vi "Text control 2 v3.4.vi"() -> ()   [LabVIEW 2016]
panel:
  out "I vs Vd":cluster{"Y data in":dbl[], "X data in":dbl[]}[](graph)
  in  "Auto Reset":bool
  in  "Reset":bool
  out "Id min vs time":cluster{"Y data in":dbl[], "X data in":dbl[]}[](graph)
  in  "Time Offset":dbl caption="Set Start Time (s)"
  out "Total lines":i32
  out "Line running":i32
  in  "byte count":u32=64
  in  "Serial End Mode for Reads":u16(ring)=2 items=["None", "LastBit", "TermChar"]
  in  "Timeout (ms)":u32=10000
  in  "Enable Termination\nChar (T)":bool=TRUE
  in  "Termination char\n(0xA = '\\n' = LF)\n(0xD = '\\r' = CR)":u8=13 format="%.0x"
  in  "flow control":u16(ring) items=["None"=0, "XON/XOFF"=1, "RTS/CTS"=2, "DTR/DSR"=4]
  in  "stop bits":u16(ring)=10 items=["1.0"=10, "1.5"=15, "2.0"=20]
  in  "parity":u16(ring) items=["None", "Odd", "Even", "Mark", "Space"]
  in  "data bits":u16=8 min=5 max=8 step=1
  in  "VISA resource name":refnum<visa-resource-name>="COM6"
  in  "baud rate":u32=9600
  out "Serial port output":string
  out "error out":errorcluster
  in  "Units":u16(ring) items=["Seconds", "Minutes", "Hours"]
  out "Elapsed Time":dbl caption="Elapsed Time (s)"
  out "Id max vs time":cluster{"Y data in":dbl[], "X data in":dbl[]}[](graph)
  out "Ig":dbl format="%.2e"
  out "Id":dbl format="%.2e"
  out "Is":dbl format="%.2e"
  out "I vs Vg":cluster{"Y data in":dbl[], "X data in":dbl[]}[](graph)
  in  "Panel Controls 2":T1={"Emergency Stop"=refnum, "TransGraph Max"=1e-05, "Text/Graph (text=false)"=TRUE, "TransGraph Min"=1e-11} {"TransGraph Min" format="%.2e"; "TransGraph Max" format="%.2e"}
  out "Command running:":string="#output s 0 0 0 -0.008 0.008 0.002"
  in  "Standby":T2
  in  "Full Reset":bool
  in  "SMU4":cluster{"on/off":bool, "Voltage":dbl} {"Voltage" min=-100.0 max=100.0 format="%.2f"}
  in  "Source/Drain Range":u8(slide)=6 max=11 scale=0.0..11.0
  in  "Source/Drain\nRange mode":u16(ring) items=["Auto", "Limited", "Fixed"]
  in  "Gate Range":u8(slide)=6 max=11 scale=0.0..11.0
  in  "Gate Range\nmode":u16(ring) items=["Auto", "Limited", "Fixed"]
  in  "Gate":T3={"Gate Start"=0.0, "Gate Stop"=2.0, "Gate Step (linear only)"=1.0, "Gate Compliance"=0.0001, "Gate PComp"=0.0, "Range mode"=0, "Range"=6} {"Range" max=11 scale=0.0..11.0; "Range mode" items=["Auto", "Limited", "Fixed"]; "Gate PComp" format="%^.2e"; "Gate Compliance" format="%^.2e"; "Gate Step (linear only)" format="%^.4e"; "Gate Stop" format="%^.4e"; "Gate Start" format="%^.4e"}
  in  "Drain 2":T4={"Drain Start"=0.0, "Drain Stop"=2.0, "Drain Compliance"=0.0001, "Drain Step"=1.0, "Drain PComp"=0.0, "Range mode"=0, "Range"=6} {"Range" max=11 scale=0.0..11.0; "Range mode" items=["Auto", "Limited", "Fixed"]; "Drain PComp" format="%^.2e"; "Drain Step" format="%^.4e"; "Drain Compliance" format="%^.2e"; "Drain Stop" format="%^.4e"; "Drain Start" format="%^.4e"}
  in  "Timings 2":T5={"integration time"=0, "Short/Long integration time"=0.00064, "hold time (sec)"=0.0, "delay time (sec)"=0.0, "Step Time (0 disables)"=0.0, "sweep method"=0, "Pulse period"=0.005, "Base voltage"=0.0, "Pulse width"=0.0005} {"Pulse width" min=0.0005 max=0.1 step=0.0001 format="%.4f"; "Base voltage" format="%^.4e"; "Pulse period" min=0.005 max=1.0 step=0.0001 format="%.4f"; "sweep method" items=["Continuous", "Pulsed"]; "Step Time (0 disables)" format="%.2f"; "delay time (sec)" format="%.4f"; "hold time (sec)" format="%.4f"; "Short/Long integration time" format="%^.0e"; "integration time" scale=0.0..2.0}
  in  "Panel Controls":T6={"Emergency Stop"=refnum, "TransGraph Max"=1e-05, "Text/Graph (text=false)"=TRUE} {"TransGraph Max" format="%.2e"}
  in  "Interrupt run":bool
  in  "Drain: Compliance":dbl=0.001 format="%.8f"
  in  "Gate: Compliance":dbl=0.001 format="%.8f"
  out "Path":path=path "C:/users/rlp38/09Apr2009LTtesting/test2.txt"
  in  "hold time /s":dbl format="%.2f"
  in  "delay time /s":dbl format="%.2f"
  in  "integration time":u32(slide) max=2 step=1 scale=0.0..2.0
  in  "Integration time (short)":dbl=0.0019 min=8e-05 max=0.0019 step=8e-05 format="%^.0e"
  in  "Integration time (long)":dbl=0.32 min=0.04 max=2.0 step=0.02 format="%.2f"
  in  "Step delay /s":dbl format="%.2f"
  in  "Program":string="#pulsedstressV d 0.03 20 0 0.5 0.0827 5\n#\n#itime s\n#gaterangemode l\n#drainrangemode l\n#pulsed on 0.05 0 0.02\n#transfer d 1 -1 -0.1 -1 -1 0\n#wait-min 1\n#transfer d 1 -1 -0.1 -1 -1 0\n#output d 0 -1 -0.5 0 -1 -0.1\n#transfer d -10 40 1 5 40 35\n#transfer d -10 40 1 5 40 35\n#output d 0 40 20 0 40 1\n#\n#\n#sample 1 0.008 221 6 0.003\n#samplei 400e-6 200 6 0.002 0.1\n#vsu2pulse -10 4\n#\n#stressV 0.016 0.03 2e-4 0.1e-3 11\n#stressI 220e-7 0.08 15\n#transfer s -1 1 0.5 -0.005 0.005 0.005\n#output s 0 0 0 -0.008 0.008 0.002\n"
  # "Serial port settings"
  # "Time"
  # "1\n2\n3\n4\n5\n6\n7\n8\n9\n10\n11\n12\n13\n14\n15\n16\n17\n18\n19\n20\n21\n22\n23\n24\n25"
  # "100 samples is approx 13s with medium integration"
  # "Syntax:\nitime [s|m|l]\ngaterangemode [a|l|f]\ndrainrangemode [a|l|f]\npulsed [on|off] PulsePeriod(sec) PulseBaseVoltage PulseONWidth(sec)\nstandby [on l off]\nwait NumMilliseconds\nwait-min NumMinutes\n# texthere = comment\ntransfer [s|d] VgStart VgStop VgStep VdStart VdStop VdStep\noutput [s|d] VgStart VgStop VgStep VdStart VdStop VdStep\nsample Vg Vd NumSamples Time(s) SampleInterval(s)\nsamplei Idg NumSamples Time(s) SampleInterval(s) VDGcompliance\n# if in doubt use SampleInterval(s) = 0.004\nstressV VG VD IGcompliance IDcompliance Duration(sec)\nstressI IDG VDGcompliance Duration(sec)\nvsu2pulse Bias Duration(s)\npulsedstressV [s|d] VEstop VgON VgOFF Period(s) PulseONwidth(s) Vd\nsample-fpp Vg Vd NumSamples Time\nresample-fpp Vg Vd\ntransfer-fpp [s|d] VgStart VgStop VgStep VdStart VdStop VdStep\noutput-fpp [s|d] VgStart VgStop VgStep VdStart VdStop VdStep\nserial SerialPortCommand"
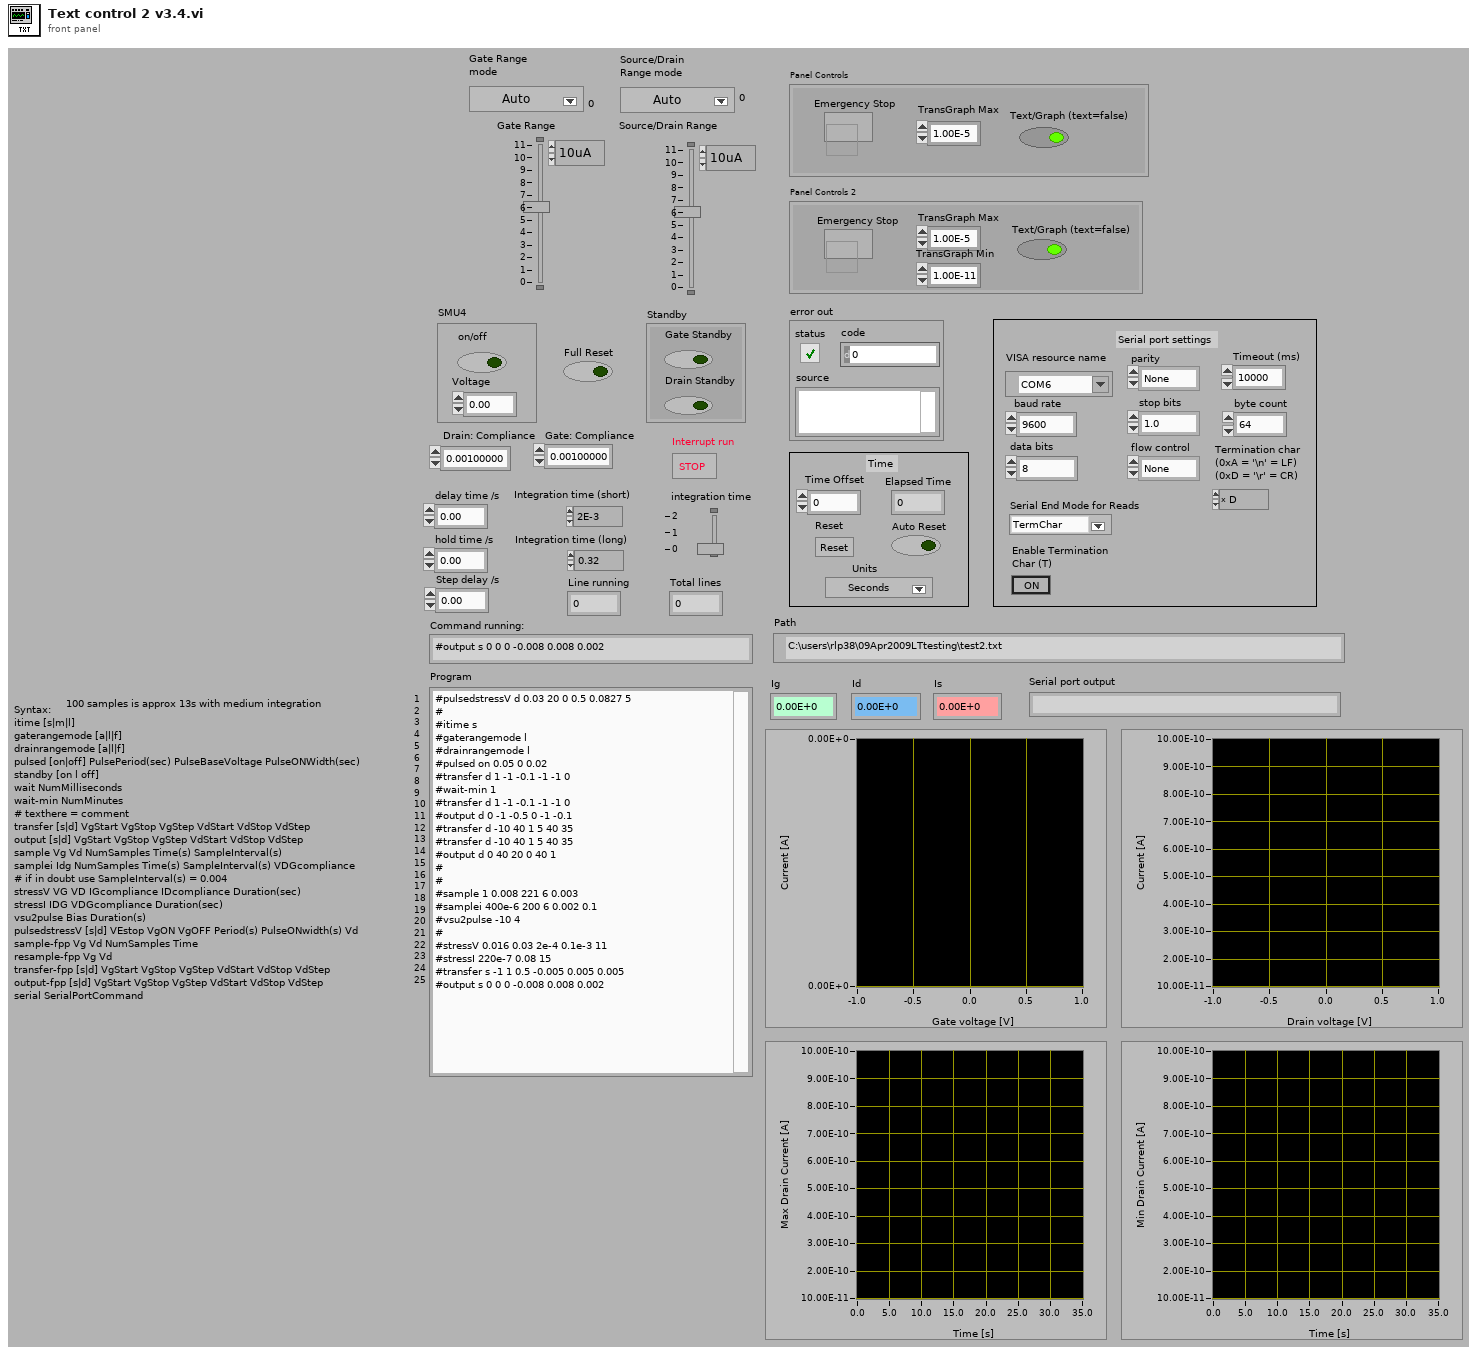
[diagram p1: front panel]
types:
  T1 = cluster{"Emergency Stop":refnum<vi>, "TransGraph Max":dbl, "Text/Graph (text=false)":bool, "TransGraph Min":dbl}
  T2 = cluster{"Gate Standby":bool, "Drain Standby":bool}
  T3 = cluster{"Gate Start":dbl, "Gate Stop":dbl, "Gate Step (linear only)":dbl, "Gate Compliance":dbl, "Gate PComp":dbl, "Range mode":u16, "Range":u8}
  T4 = cluster{"Drain Start":dbl, "Drain Stop":dbl, "Drain Compliance":dbl, "Drain Step":dbl, "Drain PComp":dbl, "Range mode":u16, "Range":u8}
  T5 = cluster{"integration time":u32, "Short/Long integration time":dbl, "hold time (sec)":dbl, "delay time (sec)":dbl, "Step Time (0 disables)":dbl, "sweep method":u16, "Pulse period":dbl, "Base voltage":dbl, "Pulse width":dbl}
  T6 = cluster{"Emergency Stop":refnum<vi>, "TransGraph Max":dbl, "Text/Graph (text=false)":bool}
  T7 = enum16{"open", "replace", "create", "open or create", "replace or create", "replace or create with confirmation"}
  T8 = cluster{"V2 Start":dbl, "V2 Step":dbl, "Number of points":i32}
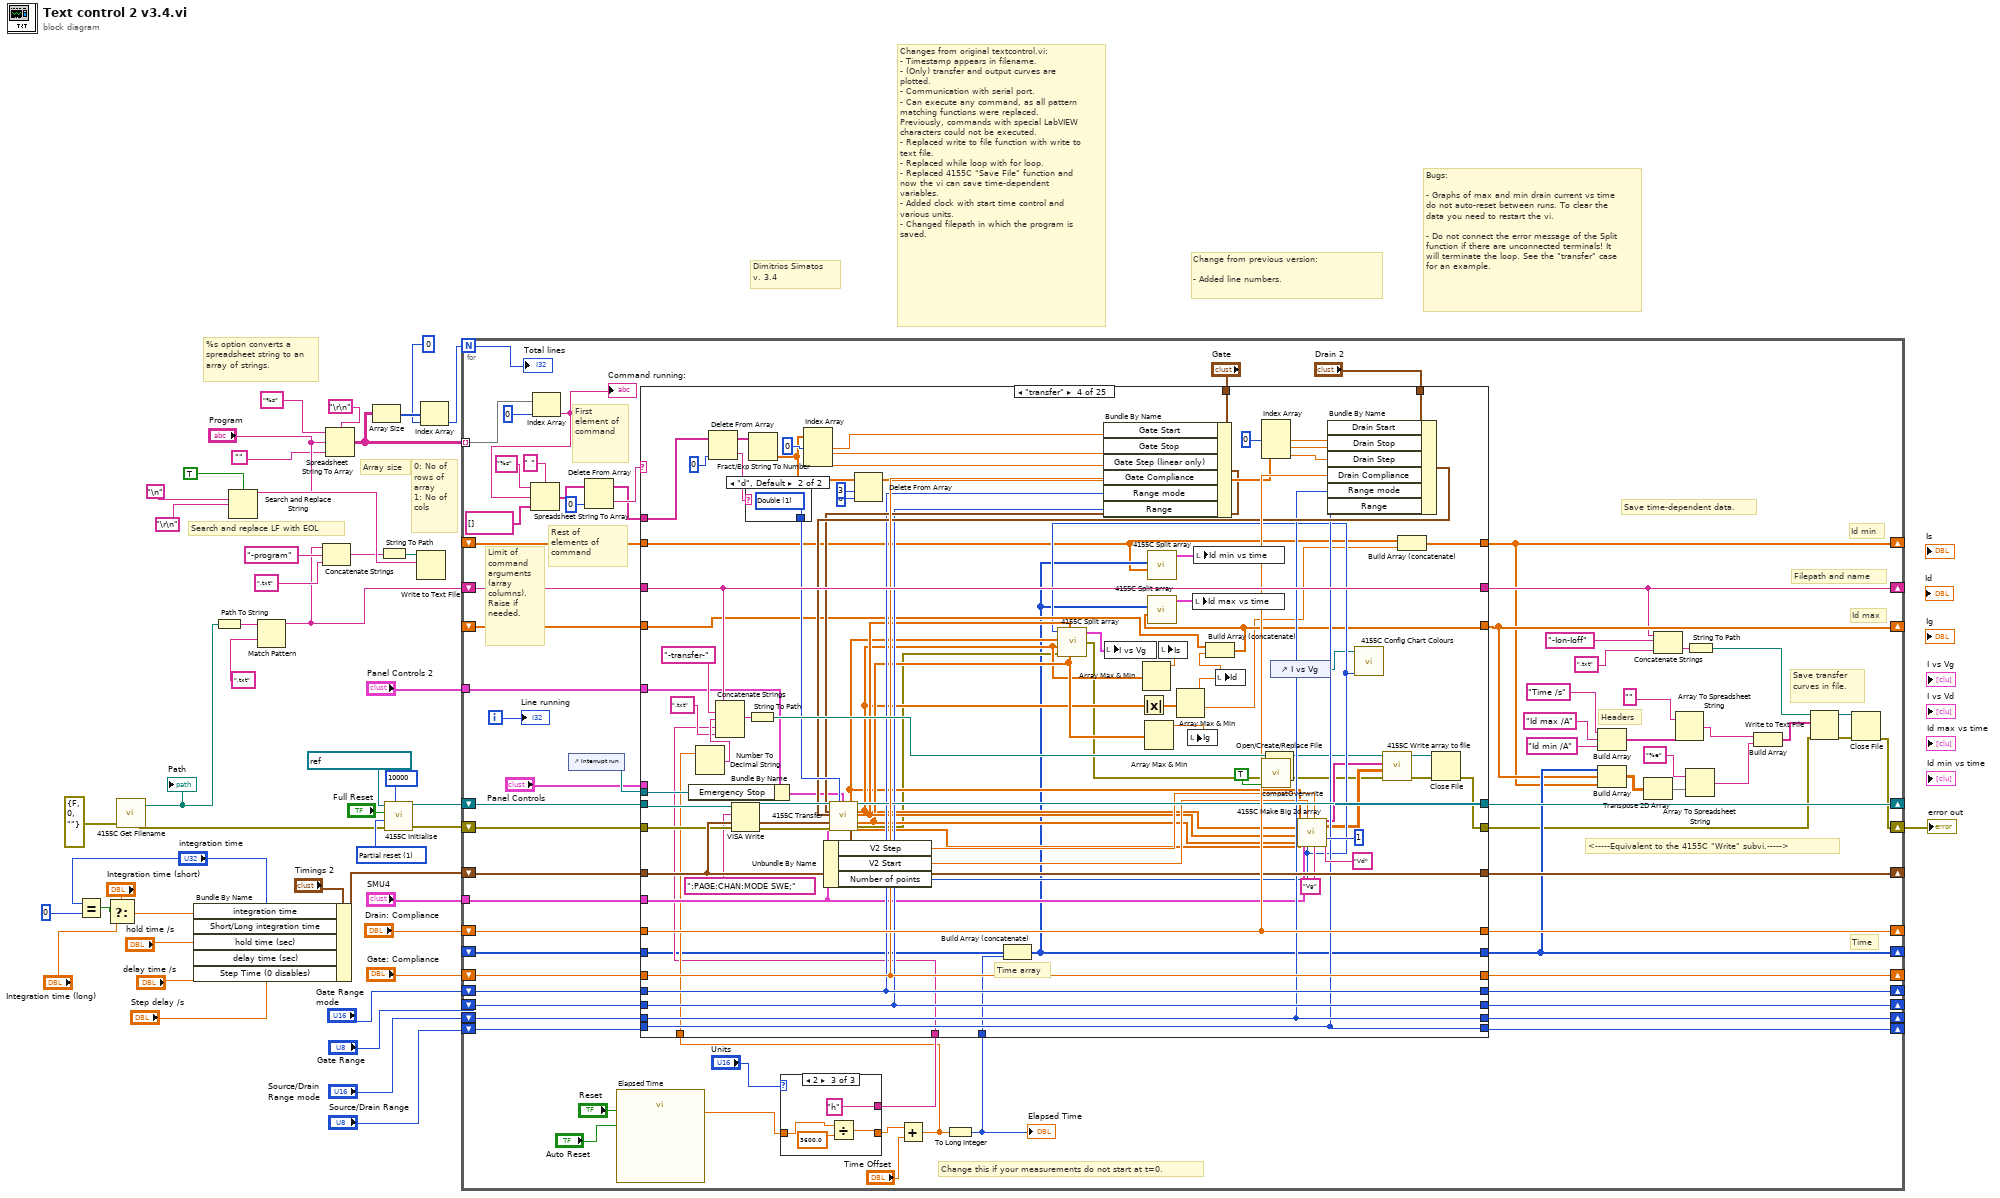
[diagram p0: block diagram]
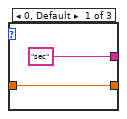
[diagram p2: hidden frame]
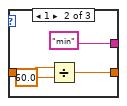
[diagram p3: hidden frame]
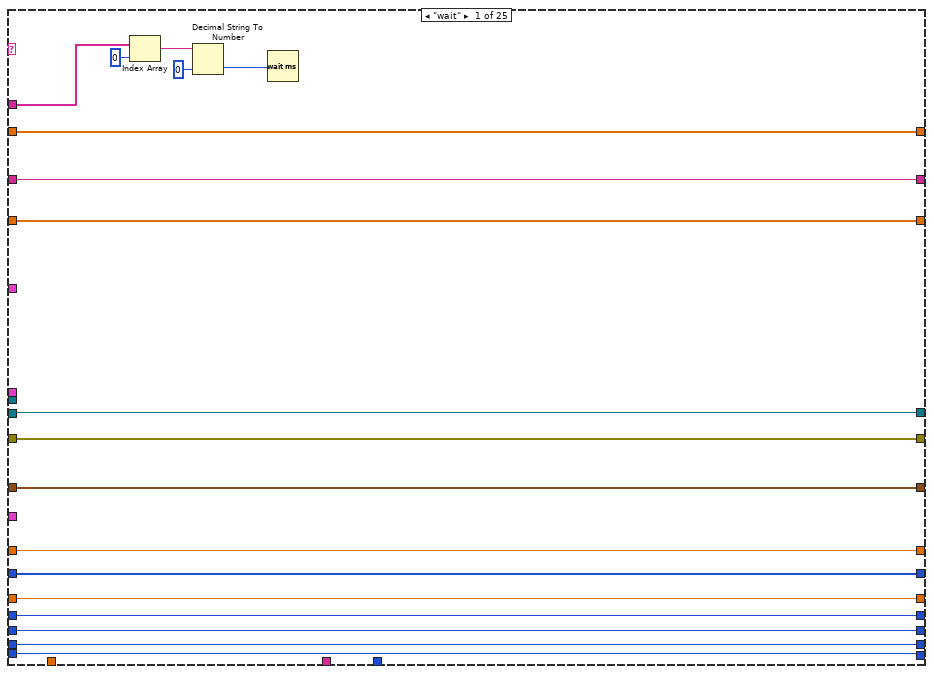
[diagram p4: hidden frame]
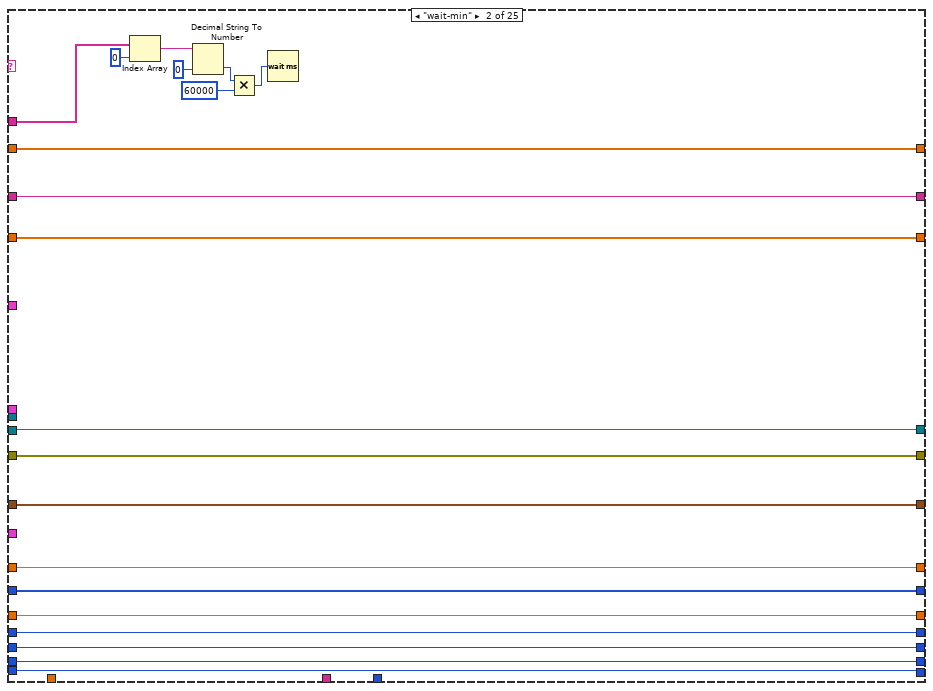
[diagram p5: hidden frame]
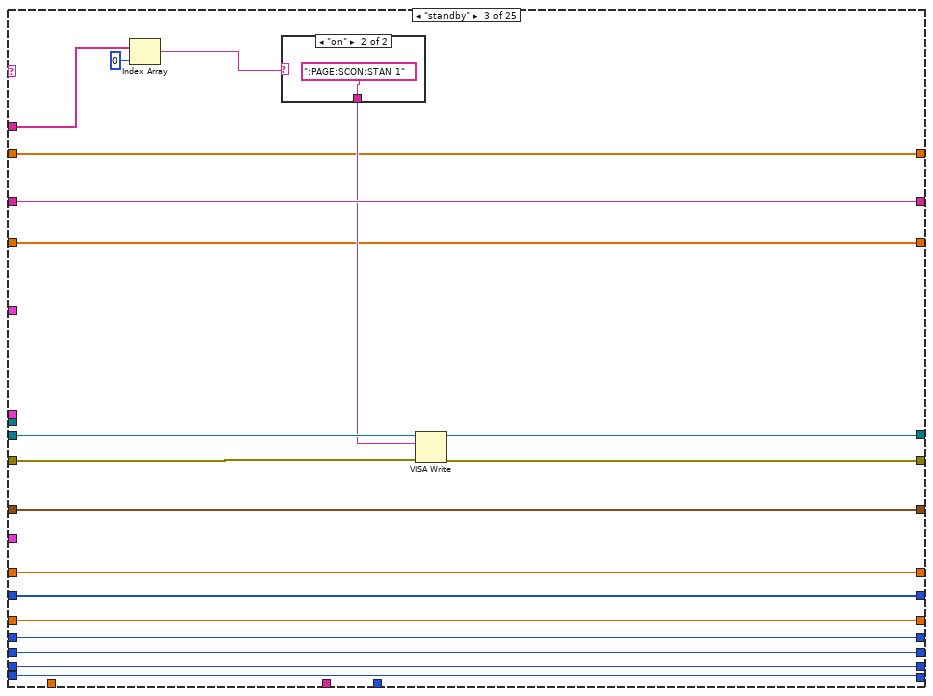
[diagram p6: hidden frame]
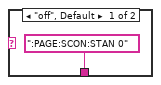
[diagram p7: hidden frame]
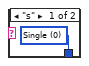
[diagram p8: hidden frame]
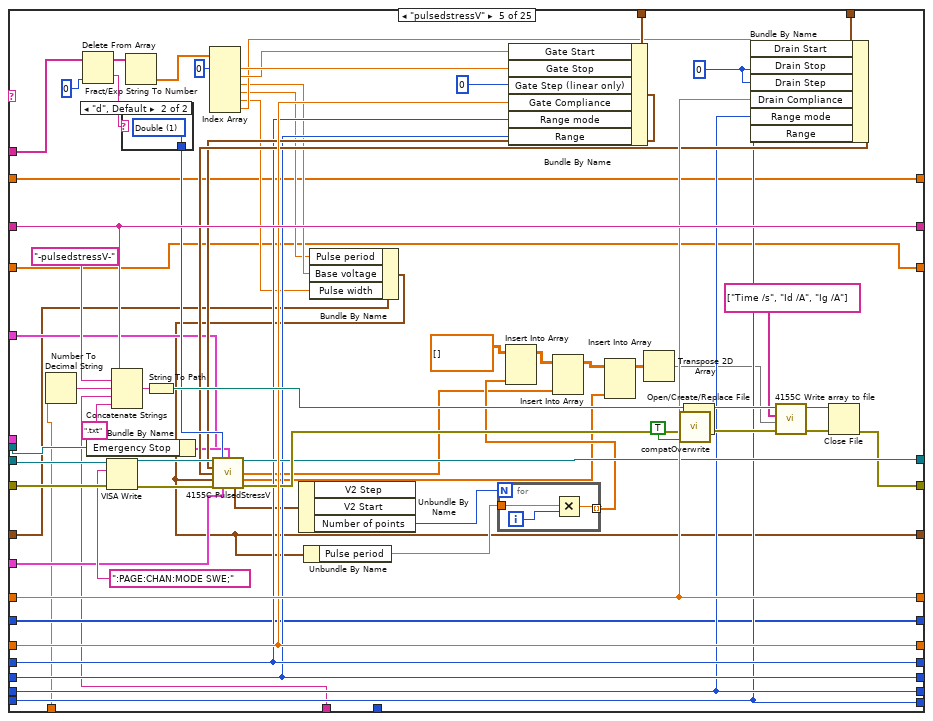
[diagram p9: hidden frame]
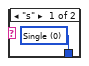
[diagram p10: hidden frame]
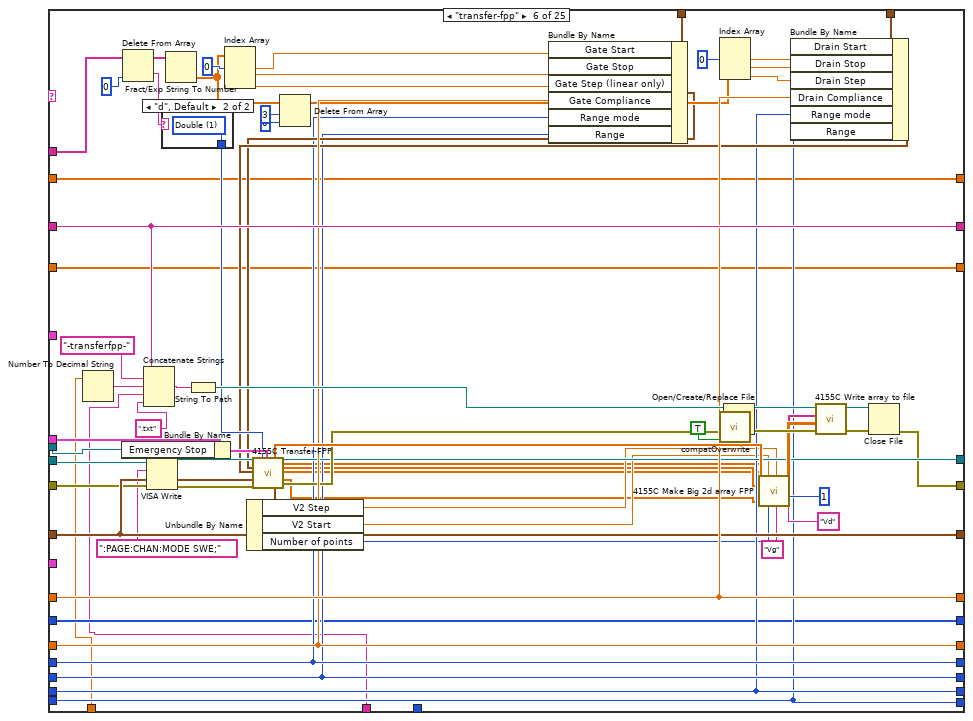
[diagram p11: hidden frame]
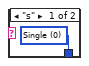
[diagram p12: hidden frame]
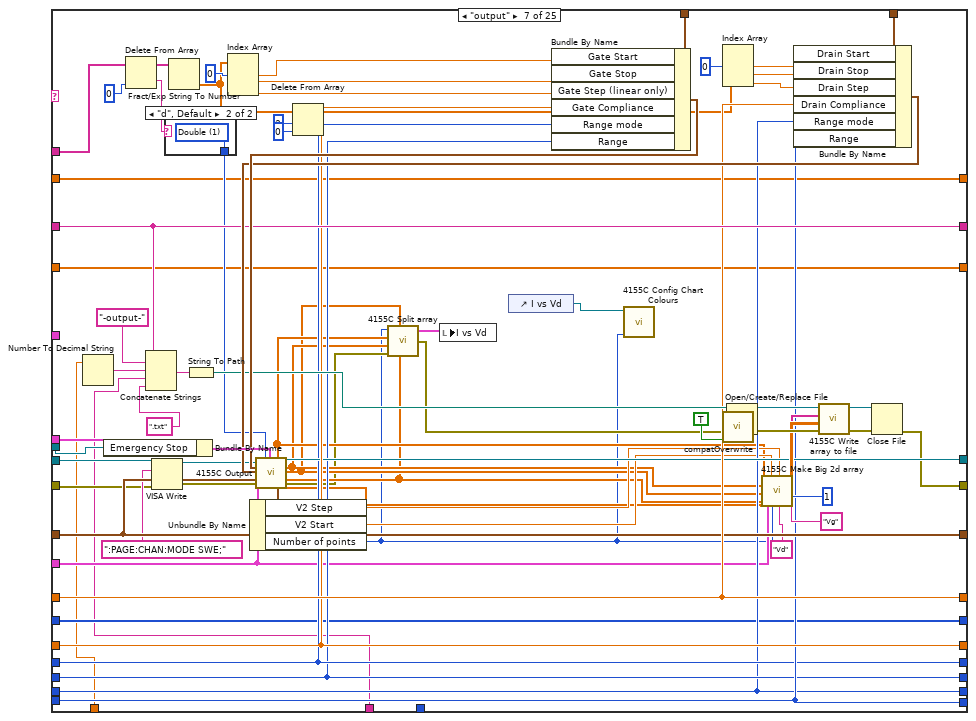
[diagram p13: hidden frame]
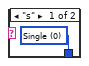
[diagram p14: hidden frame]
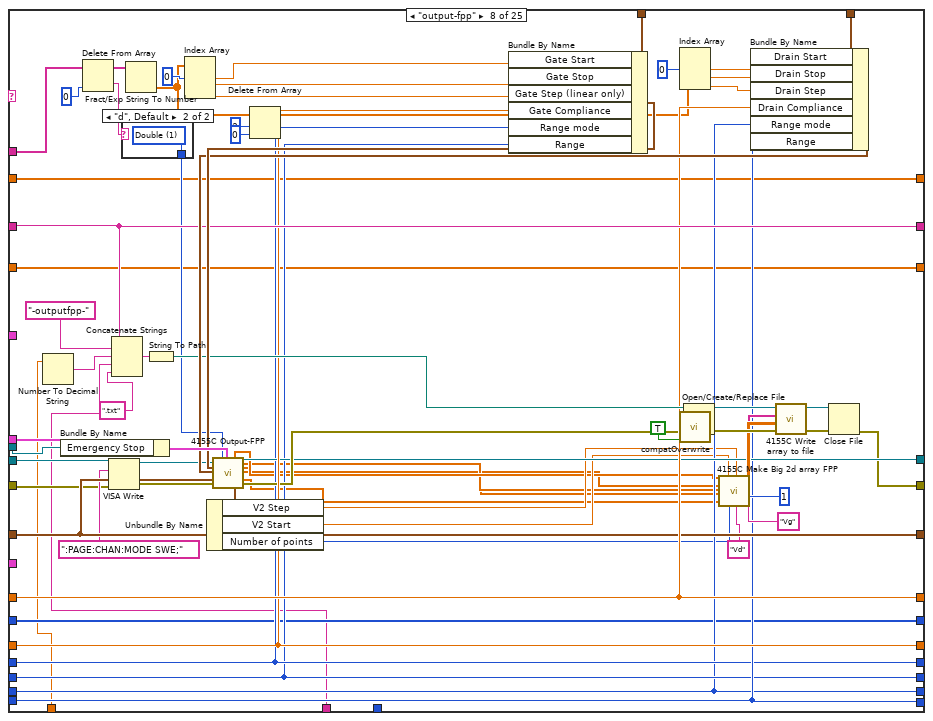
[diagram p15: hidden frame]
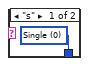
[diagram p16: hidden frame]
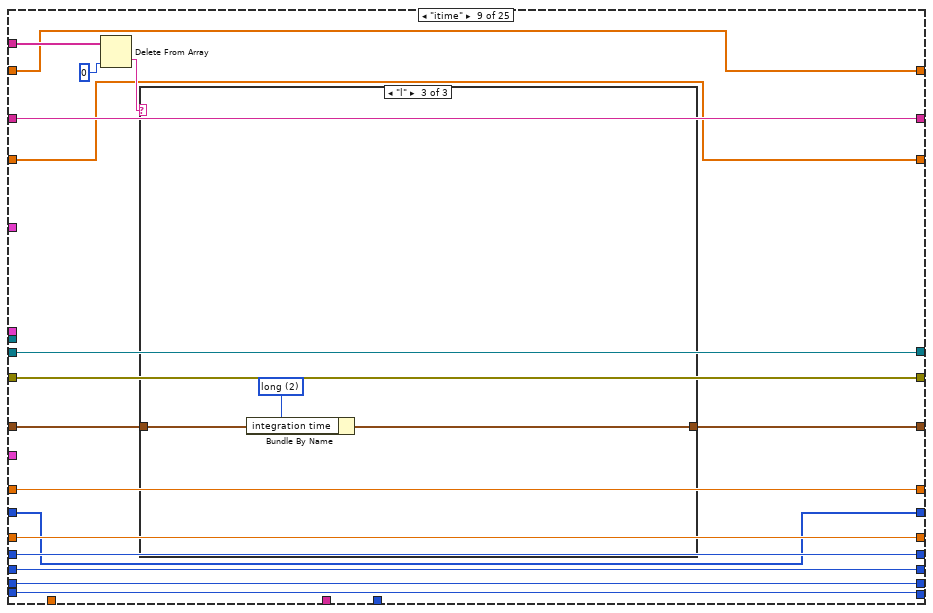
[diagram p17: hidden frame]
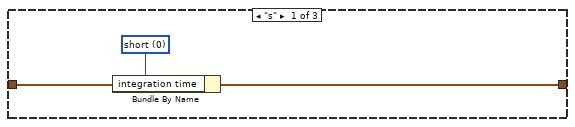
[diagram p18: hidden frame]
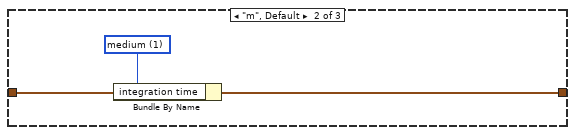
[diagram p19: hidden frame]
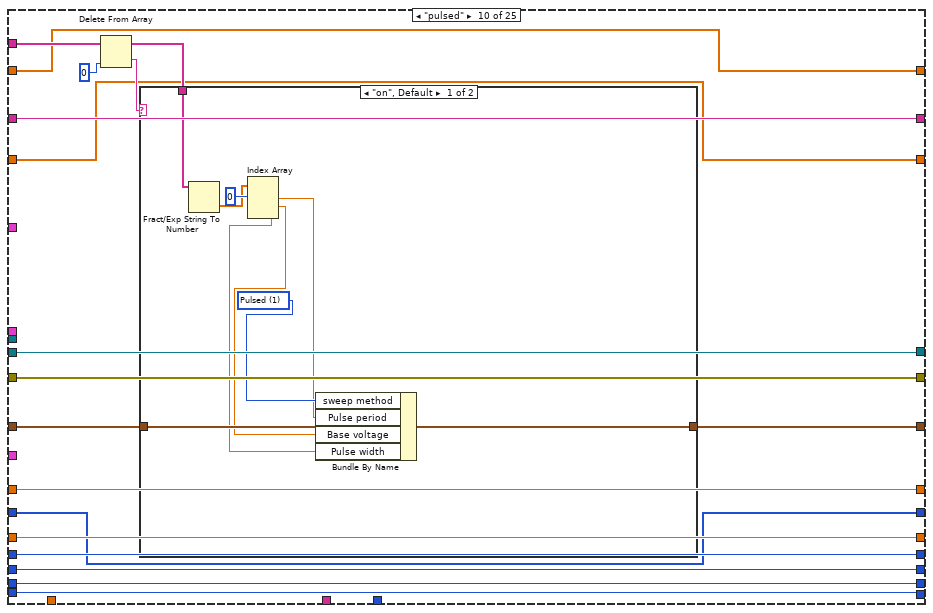
[diagram p20: hidden frame]
diagram:
  w39 = u16 1 items=["Reset All", "Partial reset"] ("Type of reset")
  # "Bugs:\n\n- Graphs of max and min drain current vs time do not auto-reset between runs. To clear the data you need to restart the vi.\n\n- Do not connect the error message of the Split function if there are unconnected terminals! It will terminate the loop. See the \"transfer\" case for an example."
  # "Array size"
  # "%s option converts a spreadsheet string to an array of strings."
  # "0: No of rows of array\n1: No of cols"
  # "Change from previous version:\n\n- Added line numbers."
  # "Dimitrios Simatos\nv. 3.4"
  # "Changes from original textcontrol.vi:\n- Timestamp appears in filename.\n- (Only) transfer and output curves are plotted.\n- Communication with serial port.\n- Can execute any command, as all pattern matching functions were replaced. Previously, commands with special LabVIEW characters could not be executed.\n- Replaced write to file function with write to text file.\n- Replaced while loop with for loop.\n- Replaced 4155C \"Save File\" function and now the vi can save time-dependent variables.\n- Added clock with start time control and various units.\n- Changed filepath in which the program is saved."
  # "Search and replace LF with EOL"
  n1 = Equal?(x="integration time", y=u32 0) -> (x = y?=w43:bool)
  n2 = Select(t="Integration time (short)", s=w43, f="Integration time (long)") -> (s? t:f=w47:dbl)
  n3 = call "4155C Get Filename.vi"("error in (no error)"=errorcluster {"status"=FALSE, "code"=0, "source"=""}) -> ("error out"=w34:errorcluster, "path"=w8:path)  [unwired: 2 in, 1 out]
  "Path" <- w8
  n4 = Bundle By Name(cluster="Timings 2", "integration time"="integration time", "Short/Long integration time"=w47, "hold time (sec)"="hold time /s", "delay time (sec)"="delay time /s", "Step Time (0 disables)"="Step delay /s") -> (w31:T5)
  n5 = Path To String(path=w8) -> (string=w9:string)
  n6 = Search and Replace String(replace all?=TRUE ("replace all? (F)"), input string="Program", search string="\n", replace string="\r\n") -> (result string=w21:string)  [unwired: 4 in, 3 out]
  n7 = Match Pattern(string=w9, regular expression=".txt") -> (before substring=w3:string)  [unwired: 1 in, 3 out]
  n8 = Concatenate Strings(w3, "-program" ("Prefix"), ".txt" ("regular expression")) -> (w2:string)
  n9 = Spreadsheet String To Array(delimiter (Tab)="\r\n", format string="%s", spreadsheet string="Program", array type (2D Dbl)="") -> (array=w12:string[][])
  n10 = Array Size(array=w12) -> (size(s)=w16:i32[])
  n11 = String To Path(string=w2) -> (path=w1:path)
  n12 = call "4155C Initialise.vi"("VISA resource name in"=refnum<visa-resource-name> "GPIB0::14::INSTR", "Reset"="Full Reset", "Type of reset"=w39, "error in (no error)"=w34, "VISA Timeout Value"=u32 10000) -> ("VISA Resource Name out"=w33:refnum<visa-resource-name>, "error out"=w32:errorcluster)
  n13 = Write to Text File(file (use dialog)=w1, text=w21) -> ()  [unwired: 2 in, 3 out]
  n14 = Index Array(array=w16, index=0) -> (element=w14:i32)
  n15 = for {
    N: w14 -> [w86]
    tunnel: "SMU4" -> [w97]
    shift-left: "Source/Drain Range" -> [w102]
    shift-right: [w98] -> _
    shift-left: "Source/Drain\nRange mode" -> [w103]
    shift-right: [w99] -> _
    shift-left: "Gate Range" -> [w104]
    shift-right: [w100] -> _
    shift-left: "Gate Range\nmode" -> [w105]
    shift-right: [w101] -> _
    shift-left: "Gate: Compliance" -> [w114]
    shift-right: [w110] -> _
    shift-left: "Drain: Compliance" -> [w115]
    shift-right: [w111] -> _
    shift-left: w31 -> [w116]
    shift-right: [w112] -> _
    shift-left: w32 -> [w117]
    shift-right: [w56] -> w7
    shift-left: w33 -> [w118]
    shift-right: [w113] -> _
    shift-left: w3 -> [w119]
    shift-right: [w59] -> _
    tunnel: "Panel Controls 2" -> [w96]
    shift-right: [w62] -> _
    shift-left: _ -> [w95]
    shift-right: [w63] -> _
    shift-left: _ -> [w91]
    tunnel: w12 -> [w89] mode=indexing
    shift-right: [w54] -> _
    shift-left: _ -> [w55]
    i -> [w87]
    # "<-----Equivalent to the 4155C \"Write\" subvi.----->"
    # "Headers"
    # "Save transfer curves in file."
    # "Filepath and name"
    # "Save time-dependent data."
    # "Change this if your measurements do not start at t=0."
    # "Time"
    # "Rest of elements of command"
    # "Id min"
    # "Id max"
    # "Limit of command arguments (array columns). Raise if needed."
    # "First element of command"
    n16 = Index Array(array=w89, index=0 ("line index")) -> (element=w82:string)
    "Command running:" <- w82
    n17 = Spreadsheet String To Array(delimiter (Tab)=" ", format string="%s", spreadsheet string=w82, array type (2D Dbl)=string[] []) -> (array=w79:string[])
    n18 = control-ref of="Interrupt run"() -> (w109:refnum<vi>)
    n19 = Delete From Array(array=w79, index=0) -> (deleted portion=w80:string, array with subset deleted=w78:string[])  [unwired: 1 in]
    n20 = call "Elapsed Time"("Reset"="Reset", "Auto Reset"="Auto Reset") -> ("Elapsed Time (s)"=w92:dbl)  [unwired: 10 in, 7 out]
    n21 = case shown="2" "Units" {
      tunnel: ["sec" "min" "h"] -> w93
      tunnel: [w120 w124 w127] -> w50
      tunnel: w92 -> [w120 w123 w128]
      frame 0, Default {
      }
      frame 1 {
        n22 = Divide(x=w123, y=60.0) -> (x/y=w124:dbl)
      }
      frame 2 {
        n23 = Divide(x=w128, y=3600.0) -> (x/y=w127:dbl)
      }
    }
    n24 = Add(x=w50, y="Time Offset") -> (x+y=w49:dbl)
    n25 = To Long Integer(number=w49) -> (32bit integer=w90:i32)
    "Elapsed Time" <- w90
    n26 = case shown="\"transfer\"" w80 {
      tunnel: w78 -> [w147 w167 w186 w262 w327 w397 w473 w544 w583 w610 w638 w664 w686 w701 _ _ w808 w870 _ w937 w982 w1025 w1096 w1159 w1167]
      tunnel: w119 -> [w142 w163 w184 w269 w334 w405 w480 w552 w572 w599 w630 w657 w680 w694 w714 w757 w786 w852 w884 w924 w969 w1013 w1090 w1155 w1169]
      tunnel: w118 -> [w141 w162 w175 w240 w318 w374 w449 w520 w573 w600 w631 w658 w681 w695 w719 w759 w814 w876 w888 w943 w988 w1031 w1102 w1113 w1173]
      tunnel: w117 -> [w140 w161 w174 w239 w317 w373 w446 w517 w574 w601 w632 w659 w682 w696 w718 w730 w813 w875 w887 w942 w987 w1030 w1101 w1112 w1172]
      tunnel: w116 -> [w139 w160 w183 w265 w293 w401 w476 w548 w582 w609 w629 w656 w679 w693 w717 w754 w777 w844 w893 w917 w962 w1006 w1089 w1154 w1174]
      tunnel: w115 -> [w138 w159 w182 w267 w332 w403 w478 w550 w581 w608 w637 w663 w685 w700 w716 w739 w812 w874 w896 w941 w986 w1029 w1100 w1163 w1175]
      tunnel: w114 -> [w137 w158 w181 w266 w331 w402 w477 w549 w580 w607 w636 w662 w684 w699 w715 w740 w787 w853 w895 w925 w970 w1014 w1091 w1156 w1177]
      tunnel: [w141 w162 w173 w264 w329 w399 w475 w546 w573 w600 w631 w658 w681 w695 w719 w759 w778 w826 w886 w918 w963 w1007 w1042 w1115 w1173] -> w113
      tunnel: [w140 w161 w172 w263 w328 w398 w474 w545 w574 w601 w632 w659 w682 w696 w718 w729 w788 w827 w885 w926 w971 w1015 w1041 w1114 w1171] -> w57
      tunnel: [w139 w160 w183 w265 w289 w401 w476 w548 w575 w602 w629 w656 w679 w693 w717 w754 w777 w844 w893 w917 w962 w1006 w1089 w1154 w1174] -> w112
      tunnel: [w138 w159 w182 w267 w332 w403 w478 w550 w581 w608 w637 w663 w685 w700 w716 w739 w812 w874 w896 w941 w986 w1029 w1100 w1163 w1175] -> w111
      tunnel: [w137 w158 w181 w266 w331 w402 w477 w549 w580 w607 w636 w662 w684 w699 w715 w740 w787 w853 w895 w925 w970 w1014 w1091 w1156 w1177] -> w110
      tunnel: [w142 w163 w184 w269 w334 w405 w480 w552 w572 w599 w630 w657 w680 w694 w714 w757 w786 w852 w884 w924 w969 w1013 w1090 w1155 w1169] -> w59
      tunnel: w109 -> [_ _ _ w272 w338 w410 w484 w556 _ _ _ _ _ _ _ _ w783 w849 _ w923 w968 w1012 w1062 w1131 _]
      tunnel: "Gate" -> [_ _ _ w249 w321 w384 w460 w531 _ _ _ _ _ _ _ _ _ _ _ _ _ _ _ _ _]
      tunnel: "Drain 2" -> [_ _ _ w248 w320 w383 w459 w530 _ _ _ _ _ _ _ _ _ _ _ _ _ _ _ _ _]
      tunnel: "Panel Controls" -> [_ _ _ _ _ w382 w458 w529 _ _ _ _ _ _ _ _ _ _ _ _ _ _ _ _ _]
      tunnel: w105 -> [w136 w157 w180 w233 w311 w367 w444 w515 w579 w606 _ w655 w678 w692 w713 w741 w773 w840 w889 w913 w958 w1002 w1085 w1150 w1178]
      tunnel: w104 -> [w135 w156 w179 w232 w310 w366 w443 w514 w578 w605 w635 _ w669 w698 w712 w742 w774 w841 w890 w914 w959 w1003 w1086 w1151 w1179]
      tunnel: w103 -> [w134 w155 w178 w231 w309 w365 w442 w513 w577 w604 w634 w661 w683 _ w711 w743 w775 w842 w891 w915 w960 w1004 w1087 w1152 w1180]
      tunnel: w102 -> [w133 w154 w177 w230 w308 w364 w445 w516 w576 w603 w633 w660 _ w697 w710 w744 w776 w843 w892 w916 w961 w1005 w1088 w1153 w1181]
      tunnel: [w136 w157 w180 w233 w311 w367 w444 w515 w579 w606 w628 w655 w678 w692 w713 w741 w773 w840 w889 w913 w958 w1002 w1085 w1150 w1178] -> w101
      tunnel: [w135 w156 w179 w232 w310 w366 w443 w514 w578 w605 w635 w647 w669 w698 w712 w742 w774 w841 w890 w914 w959 w1003 w1086 w1151 w1179] -> w100
      tunnel: [w134 w155 w178 w231 w309 w365 w442 w513 w577 w604 w634 w661 w683 w691 w711 w743 w775 w842 w891 w915 w960 w1004 w1087 w1152 w1180] -> w99
      tunnel: [w133 w154 w177 w230 w308 w364 w445 w516 w576 w603 w633 w660 w670 w697 w710 w744 w776 w843 w892 w916 w961 w1005 w1088 w1153 w1181] -> w98
      tunnel: w97 -> [_ _ _ w225 w305 _ w438 _ _ _ _ _ _ _ _ _ _ _ _ _ _ _ _ _ _]
      tunnel: w96 -> [_ _ _ w223 w304 _ _ _ _ _ _ _ _ _ _ _ _ _ _ _ _ _ _ _ _]
      tunnel: [w132 w150 w170 w200 w281 w354 w435 w502 w571 w597 w627 w646 w668 w690 w709 w725 w765 w824 w883 w902 w951 w996 w1039 w1108 w1170] -> w62
      tunnel: w95 -> [w132 w150 w170 w214 w281 w354 w435 w502 w571 w597 w627 w646 w668 w690 w709 w725 w765 w824 w883 w902 w951 w996 w1039 w1108 w1170]
      tunnel: w49 -> [_ _ _ w210 w278 w352 w432 w499 _ _ _ _ _ _ _ w723 w763 w821 _ w899 w948 w993 w1036 w1104 _]
      tunnel: w93 -> [_ _ _ w207 w277 w350 w431 w498 _ _ _ _ _ _ _ w721 w761 w820 _ w898 w947 w992 w1035 w1105 _]
      tunnel: w90 -> [_ _ _ w201 _ _ _ _ _ _ _ _ _ _ _ _ _ _ _ _ _ _ _ _ _]
      tunnel: [w131 w149 w169 w198 w280 w353 w434 w501 w570 w596 w626 w645 w667 w689 w708 w724 w764 w823 w882 w901 w950 w995 w1038 w1107 w1176] -> w63
      tunnel: w91 -> [w131 w149 w169 w206 w280 w353 w434 w501 w570 w596 w626 w645 w667 w689 w708 w724 w764 w823 w882 w901 w950 w995 w1038 w1107 w1176]
      tunnel: [w130 w148 w168 w196 w276 w349 w430 w497 w569 w595 w625 w644 w666 w688 w707 w720 w760 w819 w881 w897 w946 w991 w1034 w1103 w1164] -> w54
      tunnel: w55 -> [w130 w148 w168 w195 w276 w349 w430 w497 w569 w595 w625 w644 w666 w688 w707 w720 w760 w819 w881 w897 w946 w991 w1034 w1103 w1164]
      frame "wait" {
        n27 = Index Array(array=w147, index=0 ("Index")) -> (element=w145:string)
        n28 = Decimal String To Number(string=w145, default (0L)=u32 0) -> (number=w144:u32)  [unwired: 1 in, 1 out]
        n29 = Wait (ms)(milliseconds to wait=w144) -> ()  [unwired: 1 out]
      }
      frame "wait-min" {
        n30 = Index Array(array=w167, index=0 ("Index")) -> (element=w165:string)
        n31 = Decimal String To Number(string=w165, default (0L)=u32 0) -> (number=w153:u32)  [unwired: 1 in, 1 out]
        n32 = Multiply(x=w153, y=u32 60000) -> (x*y=w152:u32)
        n33 = Wait (ms)(milliseconds to wait=w152) -> ()  [unwired: 1 out]
      }
      frame "standby" {
        n34 = Index Array(array=w186, index=0 ("Index")) -> (element=w176:string)
        n35 = case shown="\"on\"" w176 {
          tunnel: [":PAGE:SCON:STAN 0" ":PAGE:SCON:STAN 1"] -> w171
          frame "off", Default {
          }
          frame "on" {
          }
        }
        n36 = VISA Write(VISA resource name=w175, write buffer=w171, error in (no error)=w174) -> (VISA resource name out=w173:refnum<visa-resource-name>, error out=w172:errorcluster)  [unwired: 1 out]
      }
      frame "transfer" {
        # "Time array"
        n37 = Bundle By Name(cluster=w223, "Emergency Stop"=w272) -> (w224:T1)
        n38 = Number To Decimal String(number=w210) -> (decimal integer string=w209:string)  [unwired: 1 in]
        n39 = Delete From Array(array=w262, index=0 ("Index")) -> (deleted portion=w260:string, array with subset deleted=w259:string[])  [unwired: 1 in]
        n40 = Concatenate Strings(w269, "-transfer-" ("Prefix"), w209, w207, ".txt" ("Suffix")) -> (w271:string)
        n41 = VISA Write(VISA resource name=w240, write buffer=":PAGE:CHAN:MODE SWE;" ("write buffer (\"\")"), error in (no error)=w239) -> (VISA resource name out=w237:refnum<visa-resource-name>, error out=w238:errorcluster)  [unwired: 1 out]
        n42 = case shown="\"d\", Default" w260 {
          tunnel: [w274 w275] -> w258
          frame "s" {
            w274 = u16 0 items=["Single", "Double"] ("sweep mode")
          }
          frame "d", Default {
            w275 = u16 1 items=["Single", "Double"] ("sweep mode")
          }
        }
        n43 = String To Path(string=w271) -> (path=w268:path)
        n44 = Fract/Exp String To Number(string=w259) -> (number=w244:dbl[])  [unwired: 3 in, 1 out]
        n45 = Index Array(array=w244, index #1=0 ("Index")) -> (element #1=w257:dbl, element #2=w256:dbl, element #3=w255:dbl)  [unwired: 2 in]
        n46 = Delete From Array(array=w244, length=3 ("Length"), index=0 ("Index")) -> (array with subset deleted=w242:dbl[])  [unwired: 1 out]
        n47 = Build Array (concatenate)(w206, w201) -> (w198:i32[])
        n48 = Bundle By Name(cluster=w249, "Gate Start"=w257, "Gate Stop"=w256, "Gate Step (linear only)"=w255, "Gate Compliance"=w266, "Range mode"=w233, "Range"=w232) -> (w234:T3)
        n49 = call "4155C Split array.vi"("X data in"=w198, "Y1 data in"=w195) -> ("Array of clusters"=w199:cluster{"Y data in":dbl[], "X data in":dbl[]}[])  [unwired: 5 in, 1 out]
        n50 = local write "Id min vs time"(w199) -> ()
        n51 = Index Array(array=w242, index #1=0 ("Index")) -> (element #1=w252:dbl, element #2=w251:dbl, element #3=w250:dbl)  [unwired: 2 in]
        n52 = call <vilib>:"compatOverwrite.vi"("overwrite (F)"=TRUE) -> ("overwrite?"=w222:T7)
        n53 = control-ref of="I vs Vg"() -> (w211:refnum<vi>)
        n54 = Bundle By Name(cluster=w248, "Drain Start"=w252, "Drain Stop"=w251, "Drain Step"=w250, "Drain Compliance"=w267, "Range mode"=w231, "Range"=w230) -> (w235:T4)
        n55 = call "4155C Transfer.vi"("VISA resource name in"=w237, "Gate"=w234, "Drain"=w235, "Timings"=w265, "error in (no error)"=w238, "SMU4"=w225, "sweep mode"=w258, "Panel Controls"=w224) -> ("VG"=w215:dbl[], "Outparams"=w229:T8, "VISA Resource Name out"=w264:refnum<visa-resource-name>, "IS"=w216:dbl[], "ID"=w221:dbl[], "IG"=w217:dbl[], "error out"=w202:errorcluster, "SMU4"=w226:dbl[])  [unwired: 12 in]
        n56 = Unbundle By Name(w229) -> ("V2 Step"=w228:dbl, "V2 Start"=w227:dbl, "Number of points"=w212:i32)
        n57 = call "4155C Split array.vi"("Number of VAR2 steps"=w212, "Y2 data in"=w221, "X data in"=w215, "Y1 data in"=w216, "Y3 data in"=w217, "error in (no error)"=w202) -> ("Array of clusters"=w205:cluster{"Y data in":dbl[], "X data in":dbl[]}[], "error out"=w203:errorcluster)  [unwired: 1 in]
        n58 = local write "I vs Vg"(w205) -> ()
        n59 = Absolute Value(x=w216) -> (abs(x)=w220:dbl[])
        n60 = Array Max & Min(array=w216) -> (max value=w218:dbl)  [unwired: 3 out]
        n61 = Array Max & Min(array=w217) -> (max value=w219:dbl)  [unwired: 3 out]
        n62 = local write "Is"(w218) -> ()
        n63 = Array Max & Min(array=w220) -> (max value=w213:dbl, min value=w197:dbl)  [unwired: 2 out]
        n64 = local write "Ig"(w219) -> ()
        n65 = Build Array (concatenate)(w214, w213) -> (w200:dbl[])
        n66 = call "4155C Split array.vi"("X data in"=w198, "Y1 data in"=w200) -> ("Array of clusters"=w204:cluster{"Y data in":dbl[], "X data in":dbl[]}[])  [unwired: 5 in, 1 out]
        n67 = local write "Id max vs time"(w204) -> ()
        n68 = local write "Id"(w213) -> ()
        n69 = Open/Create/Replace File(file path (use dialog)=w268, error in=w203, operation (0:open)=w222) -> (refnum out=w193:refnum<file>, error out=w191:errorcluster)  [unwired: 3 in, 1 out]
        n70 = call "4155C Make Big 2d array.vi"("1D Var1"=w215, "1d IS"=w216, "1d ID"=w221, "1d IG"=w217, "1d SMU4"=w226, "SMU4"=w225, "VAR2 START"=w227, "Number of VAR2 steps"=w212, "VAR2 STEP"=w228, "VAR1 Name"="Vg", "Decimal places in header"=i8 1, "VAR2 Name"="Vd") -> ("Header array"=w194:string[], "Data array"=w192:dbl[][])  [unwired: 14 in]
        n71 = call "4155C Config Chart Colours.vi"("Numeric"=w212, "XY Graph 2"=w211) -> ()  [unwired: 6 in]
        n72 = call "4155C Write array to file.vi"("Byte Stream File Refnum"=w193, "Header"=w194, "Data Array"=w192, "error in (no error)"=w191) -> ("dup refnum"=w190:refnum<file>, "error out"=w189:errorcluster)  [unwired: 1 in]
        n73 = Build Array (concatenate)(w195, w197) -> (w196:dbl[])
        n74 = Close File(refnum=w190, error in=w189) -> (error out=w263:errorcluster)  [unwired: 1 out]
      }
      frame "pulsedstressV" {
        w287 = 0
        n75 = Number To Decimal String(number=w278) -> (decimal integer string=w335:string)  [unwired: 1 in]
        n76 = Delete From Array(array=w327, index=0 ("Index")) -> (deleted portion=w325:string, array with subset deleted=w324:string[])  [unwired: 1 in]
        n77 = Bundle By Name(cluster=w304, "Emergency Stop"=w338) -> (w306:T1)
        n78 = VISA Write(VISA resource name=w318, write buffer=":PAGE:CHAN:MODE SWE;" ("write buffer (\"\")"), error in (no error)=w317) -> (VISA resource name out=w315:refnum<visa-resource-name>, error out=w316:errorcluster)  [unwired: 1 out]
        n79 = Concatenate Strings(w334, "-pulsedstressV-" ("Substring"), w335, w277, ".txt" ("Substring")) -> (w337:string)
        n80 = case shown="\"d\", Default" w325 {
          tunnel: [w347 w348] -> w323
          frame "s" {
            w347 = u16 0 items=["Single", "Double"] ("sweep mode")
          }
          frame "d", Default {
            w348 = u16 1 items=["Single", "Double"] ("sweep mode")
          }
        }
        n81 = Fract/Exp String To Number(string=w324) -> (number=w319:dbl[])  [unwired: 3 in, 1 out]
        n82 = String To Path(string=w337) -> (path=w333:path)
        n83 = Index Array(array=w319, index #1=0 ("Index")) -> (element #1=w296:dbl, element #2=w295:dbl, element #3=w292:dbl, element #4=w291:dbl, element #5=w290:dbl, element #6=w294:dbl)  [unwired: 5 in]
        n84 = Bundle By Name(cluster=w293, "Pulse period"=w291, "Base voltage"=w292, "Pulse width"=w290) -> (w289:T5)
        n85 = Unbundle By Name(w289) -> ("Pulse period"=w297:dbl)
        n86 = Bundle By Name(cluster=w321, "Gate Start"=w295, "Gate Stop"=w296, "Gate Step (linear only)"=0, "Gate Compliance"=w331, "Range mode"=w311, "Range"=w310) -> (w312:T3)
        n87 = call <vilib>:"compatOverwrite.vi"("overwrite (F)"=TRUE) -> ("overwrite?"=w282:T7)
        n88 = Bundle By Name(cluster=w320, "Drain Start"=w294, "Drain Stop"=w287, "Drain Step"=w287, "Drain Compliance"=w332, "Range mode"=w309, "Range"=w308) -> (w313:T4)
        n89 = call "4155C PulsedStressV.vi"("VISA resource name in"=w315, "sweep mode"=w323, "Panel Controls"=w306, "Gate"=w312, "Drain"=w313, "Timings"=w289, "error in (no error)"=w316, "SMU4"=w305) -> ("VISA Resource Name out"=w329:refnum<visa-resource-name>, "ID"=w285:dbl[], "IG"=w283:dbl[], "Outparams"=w307:T8, "error out"=w330:errorcluster)  [unwired: 3 in]
        n90 = Unbundle By Name(w307) -> ("Number of points"=w284:i32)  [unwired: 2 out]
        n91 = for {
          N: w284 -> [_]
          tunnel: [w344] -> w286 mode=indexing
          tunnel: w297 -> [w346]
          i -> [w345]
          n92 = Multiply(x=w346, y=w345) -> (x*y=w344:dbl)
        }
        n93 = Insert Into Array(array=dbl[][] [] ("Input Array"), new element=w286) -> (w298:dbl[][])  [unwired: 2 in]
        n94 = Insert Into Array(array=w298, new element=w285) -> (w303:dbl[][])  [unwired: 2 in]
        n95 = Insert Into Array(array=w303, new element=w283) -> (w302:dbl[][])  [unwired: 2 in]
        n96 = Transpose 2D Array(2D array=w302) -> (transposed array=w301:dbl[][])
        n97 = Open/Create/Replace File(file path (use dialog)=w333, error in=w330, operation (0:open)=w282) -> (refnum out=w341:refnum<file>, error out=w342:errorcluster)  [unwired: 3 in, 1 out]
        n98 = call "4155C Write array to file.vi"("Byte Stream File Refnum"=w341, "Header"=string[] ["Time /s", "Id /A", "Ig /A"], "Data Array"=w301, "error in (no error)"=w342) -> ("dup refnum"=w339:refnum<file>, "error out"=w340:errorcluster)  [unwired: 1 in]
        n99 = Close File(refnum=w339, error in=w340) -> (error out=w328:errorcluster)  [unwired: 1 out]
      }
      frame "transfer-fpp" {
        n100 = Number To Decimal String(number=w352) -> (decimal integer string=w406:string)  [unwired: 1 in]
        n101 = Bundle By Name(cluster=w382, "Emergency Stop"=w410) -> (w418:T6)
        n102 = Delete From Array(array=w397, index=0 ("Index")) -> (deleted portion=w395:string, array with subset deleted=w394:string[])  [unwired: 1 in]
        n103 = Concatenate Strings(w405, "-transferfpp-" ("Substring"), w406, w350, ".txt" ("Substring")) -> (w408:string)
        n104 = VISA Write(VISA resource name=w374, write buffer=":PAGE:CHAN:MODE SWE;" ("write buffer (\"\")"), error in (no error)=w373) -> (VISA resource name out=w371:refnum<visa-resource-name>, error out=w372:errorcluster)  [unwired: 1 out]
        n105 = case shown="\"d\", Default" w395 {
          tunnel: [w419 w420] -> w393
          frame "s" {
            w419 = u16 0 items=["Single", "Double"] ("sweep mode")
          }
          frame "d", Default {
            w420 = u16 1 items=["Single", "Double"] ("sweep mode")
          }
        }
        n106 = Fract/Exp String To Number(string=w394) -> (number=w378:dbl[])  [unwired: 3 in, 1 out]
        n107 = String To Path(string=w408) -> (path=w404:path)
        n108 = Index Array(array=w378, index #1=0 ("Index")) -> (element #1=w392:dbl, element #2=w391:dbl, element #3=w390:dbl)  [unwired: 2 in]
        n109 = Delete From Array(array=w378, length=3 ("Length"), index=0 ("Index")) -> (array with subset deleted=w376:dbl[])  [unwired: 1 out]
        n110 = Bundle By Name(cluster=w384, "Gate Start"=w392, "Gate Stop"=w391, "Gate Step (linear only)"=w390, "Gate Compliance"=w402, "Range mode"=w367, "Range"=w366) -> (w368:T3)
        n111 = Index Array(array=w376, index #1=0 ("Index")) -> (element #1=w387:dbl, element #2=w386:dbl, element #3=w385:dbl)  [unwired: 2 in]
        n112 = call <vilib>:"compatOverwrite.vi"("overwrite (F)"=TRUE) -> ("overwrite?"=w355:T7)
        n113 = Bundle By Name(cluster=w383, "Drain Start"=w387, "Drain Stop"=w386, "Drain Step"=w385, "Drain Compliance"=w403, "Range mode"=w365, "Range"=w364) -> (w369:T4)
        n114 = call "4155C Transfer-FPP.vi"("VISA resource name in"=w371, "Gate"=w368, "Drain"=w369, "Timings"=w401, "error in (no error)"=w372, "sweep mode"=w393, "Panel Controls"=w418) -> ("VG"=w409:dbl[], "Outparams"=w363:T8, "VISA Resource Name out"=w399:refnum<visa-resource-name>, "Vprobe2"=w359:dbl[], "ID"=w358:dbl[], "IG"=w357:dbl[], "Vprobe1"=w356:dbl[], "error out"=w400:errorcluster)  [unwired: 13 in]
        n115 = Unbundle By Name(w363) -> ("V2 Step"=w362:dbl, "V2 Start"=w361:dbl, "Number of points"=w360:i32)
        n116 = Open/Create/Replace File(file path (use dialog)=w404, error in=w400, operation (0:open)=w355) -> (refnum out=w415:refnum<file>, error out=w416:errorcluster)  [unwired: 3 in, 1 out]
        n117 = call "4155C Make Big 2d array FPP.vi"("1D Var1"=w409, "1d ID"=w358, "1d Vp2"=w359, "1d IG"=w357, "1d Vp1"=w356, "VAR2 START"=w361, "Number of VAR2 steps"=w360, "VAR2 STEP"=w362, "VAR1 Name"="Vg", "Decimal places in header"=i8 1, "VAR2 Name"="Vd") -> ("Header array"=w411:string[], "Data array"=w412:dbl[][])  [unwired: 15 in]
        n118 = call "4155C Write array to file.vi"("Byte Stream File Refnum"=w415, "Header"=w411, "Data Array"=w412, "error in (no error)"=w416) -> ("dup refnum"=w413:refnum<file>, "error out"=w414:errorcluster)  [unwired: 1 in]
        n119 = Close File(refnum=w413, error in=w414) -> (error out=w398:errorcluster)  [unwired: 1 out]
      }
      frame "output" {
        n120 = Number To Decimal String(number=w432) -> (decimal integer string=w481:string)  [unwired: 1 in]
        n121 = Bundle By Name(cluster=w458, "Emergency Stop"=w484) -> (w494:T6)
        n122 = Delete From Array(array=w473, index=0 ("Index")) -> (deleted portion=w471:string, array with subset deleted=w470:string[])  [unwired: 1 in]
        n123 = Concatenate Strings(w480, "-output-" ("Substring"), w481, w431, ".txt" ("Substring")) -> (w483:string)
        n124 = VISA Write(VISA resource name=w449, write buffer=":PAGE:CHAN:MODE SWE;" ("write buffer (\"\")"), error in (no error)=w446) -> (VISA resource name out=w448:refnum<visa-resource-name>, error out=w447:errorcluster)  [unwired: 1 out]
        n125 = case shown="\"d\", Default" w471 {
          tunnel: [w495 w496] -> w469
          frame "s" {
            w495 = u16 0 items=["Single", "Double"] ("sweep mode")
          }
          frame "d", Default {
            w496 = u16 1 items=["Single", "Double"] ("sweep mode")
          }
        }
        n126 = Fract/Exp String To Number(string=w470) -> (number=w452:dbl[])  [unwired: 3 in, 1 out]
        n127 = String To Path(string=w483) -> (path=w479:path)
        n128 = Index Array(array=w452, index #1=0 ("Index")) -> (element #1=w468:dbl, element #2=w467:dbl, element #3=w466:dbl)  [unwired: 2 in]
        n129 = Delete From Array(array=w452, length=3 ("Length"), index=0 ("Index")) -> (array with subset deleted=w451:dbl[])  [unwired: 1 out]
        n130 = control-ref of="I vs Vd"() -> (w422:refnum<vi>)
        n131 = Bundle By Name(cluster=w460, "Gate Start"=w468, "Gate Stop"=w467, "Gate Step (linear only)"=w466, "Gate Compliance"=w477, "Range mode"=w444, "Range"=w443) -> (w493:T3)
        n132 = Index Array(array=w451, index #1=0 ("Index")) -> (element #1=w463:dbl, element #2=w462:dbl, element #3=w461:dbl)  [unwired: 2 in]
        n133 = call <vilib>:"compatOverwrite.vi"("overwrite (F)"=TRUE) -> ("overwrite?"=w436:T7)
        n134 = Bundle By Name(cluster=w459, "Drain Start"=w463, "Drain Stop"=w462, "Drain Step"=w461, "Drain Compliance"=w478, "Range mode"=w442, "Range"=w445) -> (w492:T4)
        n135 = call "4155C Output.vi"("VISA resource name in"=w448, "Gate"=w493, "Drain"=w492, "Timings"=w476, "error in (no error)"=w447, "SMU4"=w438, "sweep mode"=w469, "Panel controls"=w494) -> ("VD"=w429:dbl[], "Outparams"=w440:T8, "VISA Resource Name out"=w475:refnum<visa-resource-name>, "IS"=w428:dbl[], "ID"=w427:dbl[], "IG"=w426:dbl[], "error out"=w424:errorcluster, "SMU4"=w437:dbl[])  [unwired: 12 in]
        n136 = Unbundle By Name(w440) -> ("V2 Step"=w441:dbl, "V2 Start"=w439:dbl, "Number of points"=w421:i32)
        n137 = call "4155C Split array.vi"("Number of VAR2 steps"=w421, "Y2 data in"=w427, "X data in"=w429, "Y1 data in"=w428, "Y3 data in"=w426, "error in (no error)"=w424) -> ("Array of clusters"=w425:cluster{"Y data in":dbl[], "X data in":dbl[]}[], "error out"=w423:errorcluster)  [unwired: 1 in]
        n138 = local write "I vs Vd"(w425) -> ()
        n139 = call "4155C Config Chart Colours.vi"("Numeric"=w421, "XY Graph 2"=w422) -> ()  [unwired: 6 in]
        n140 = Open/Create/Replace File(file path (use dialog)=w479, error in=w423, operation (0:open)=w436) -> (refnum out=w489:refnum<file>, error out=w490:errorcluster)  [unwired: 3 in, 1 out]
        n141 = call "4155C Make Big 2d array.vi"("1D Var1"=w429, "1d IS"=w428, "1d ID"=w427, "1d IG"=w426, "1d SMU4"=w437, "SMU4"=w438, "VAR2 START"=w439, "Number of VAR2 steps"=w421, "VAR2 STEP"=w441, "VAR1 Name"="Vd", "Decimal places in header"=i8 1, "VAR2 Name"="Vg") -> ("Header array"=w485:string[], "Data array"=w486:dbl[][])  [unwired: 14 in]
        n142 = call "4155C Write array to file.vi"("Byte Stream File Refnum"=w489, "Header"=w485, "Data Array"=w486, "error in (no error)"=w490) -> ("dup refnum"=w487:refnum<file>, "error out"=w488:errorcluster)  [unwired: 1 in]
        n143 = Close File(refnum=w487, error in=w488) -> (error out=w474:errorcluster)  [unwired: 1 out]
      }
      frame "output-fpp" {
        n144 = Number To Decimal String(number=w499) -> (decimal integer string=w553:string)  [unwired: 1 in]
        n145 = Bundle By Name(cluster=w529, "Emergency Stop"=w556) -> (w566:T6)
        n146 = Delete From Array(array=w544, index=0 ("Index")) -> (deleted portion=w542:string, array with subset deleted=w541:string[])  [unwired: 1 in]
        n147 = VISA Write(VISA resource name=w520, write buffer=":PAGE:CHAN:MODE SWE;" ("write buffer (\"\")"), error in (no error)=w517) -> (VISA resource name out=w519:refnum<visa-resource-name>, error out=w518:errorcluster)  [unwired: 1 out]
        n148 = Concatenate Strings(w552, "-outputfpp-" ("Substring"), w553, w498, ".txt" ("Substring")) -> (w555:string)
        n149 = case shown="\"d\", Default" w542 {
          tunnel: [w567 w568] -> w540
          frame "s" {
            w567 = u16 0 items=["Single", "Double"] ("sweep mode")
          }
          frame "d", Default {
            w568 = u16 1 items=["Single", "Double"] ("sweep mode")
          }
        }
        n150 = Fract/Exp String To Number(string=w541) -> (number=w523:dbl[])  [unwired: 3 in, 1 out]
        n151 = String To Path(string=w555) -> (path=w551:path)
        n152 = Index Array(array=w523, index #1=0 ("Index")) -> (element #1=w539:dbl, element #2=w538:dbl, element #3=w537:dbl)  [unwired: 2 in]
        n153 = Delete From Array(array=w523, length=3 ("Length"), index=0 ("Index")) -> (array with subset deleted=w522:dbl[])  [unwired: 1 out]
        n154 = Bundle By Name(cluster=w531, "Gate Start"=w539, "Gate Stop"=w538, "Gate Step (linear only)"=w537, "Gate Compliance"=w549, "Range mode"=w515, "Range"=w514) -> (w565:T3)
        n155 = Index Array(array=w522, index #1=0 ("Index")) -> (element #1=w534:dbl, element #2=w533:dbl, element #3=w532:dbl)  [unwired: 2 in]
        n156 = call <vilib>:"compatOverwrite.vi"("overwrite (F)"=TRUE) -> ("overwrite?"=w503:T7)
        n157 = Bundle By Name(cluster=w530, "Drain Start"=w534, "Drain Stop"=w533, "Drain Step"=w532, "Drain Compliance"=w550, "Range mode"=w513, "Range"=w516) -> (w564:T4)
        n158 = call "4155C Output-FPP.vi"("VISA resource name in"=w519, "Gate"=w565, "Drain"=w564, "Timings"=w548, "error in (no error)"=w518, "sweep mode"=w540, "Panel controls"=w566) -> ("VD"=w508:dbl[], "Outparams"=w511:T8, "VISA Resource Name out"=w546:refnum<visa-resource-name>, "Vprobe2"=w507:dbl[], "ID"=w506:dbl[], "IG"=w505:dbl[], "Vprobe1"=w504:dbl[], "error out"=w547:errorcluster)  [unwired: 13 in]
        n159 = Unbundle By Name(w511) -> ("V2 Step"=w512:dbl, "V2 Start"=w510:dbl, "Number of points"=w509:i32)
        n160 = Open/Create/Replace File(file path (use dialog)=w551, error in=w547, operation (0:open)=w503) -> (refnum out=w561:refnum<file>, error out=w562:errorcluster)  [unwired: 3 in, 1 out]
        n161 = call "4155C Make Big 2d array FPP.vi"("1D Var1"=w508, "1d ID"=w506, "1d Vp2"=w507, "1d IG"=w505, "1d Vp1"=w504, "VAR2 START"=w510, "Number of VAR2 steps"=w509, "VAR2 STEP"=w512, "VAR1 Name"="Vd", "Decimal places in header"=i8 1, "VAR2 Name"="Vg") -> ("Header array"=w557:string[], "Data array"=w558:dbl[][])  [unwired: 15 in]
        n162 = call "4155C Write array to file.vi"("Byte Stream File Refnum"=w561, "Header"=w557, "Data Array"=w558, "error in (no error)"=w562) -> ("dup refnum"=w559:refnum<file>, "error out"=w560:errorcluster)  [unwired: 1 in]
        n163 = Close File(refnum=w559, error in=w560) -> (error out=w545:errorcluster)  [unwired: 1 out]
      }
      frame "itime" {
        n164 = Delete From Array(array=w583, index=0 ("Index")) -> (deleted portion=w584:string)  [unwired: 1 in, 1 out]
        n165 = case shown="\"l\"" w584 {
          tunnel: w582 -> [w588 w590 w593]
          tunnel: [w587 w589 w592] -> w575
          frame "s" {
            w586 = u32 0 items=["short  ", "medium  ", "long  "] ("integration time 2")
            n166 = Bundle By Name(cluster=w588, "integration time"=w586) -> (w587:T5)
          }
          frame "m", Default {
            w591 = u32 1 items=["short  ", "medium  ", "long  "] ("integration time 2")
            n167 = Bundle By Name(cluster=w590, "integration time"=w591) -> (w589:T5)
          }
          frame "l" {
            w594 = u32 2 items=["short  ", "medium  ", "long  "] ("integration time 2")
            n168 = Bundle By Name(cluster=w593, "integration time"=w594) -> (w592:T5)
          }
        }
      }
      frame "pulsed" {
        n169 = Delete From Array(array=w610, index=0 ("Index")) -> (deleted portion=w611:string, array with subset deleted=w598:string[])  [unwired: 1 in]
        n170 = case shown="\"on\", Default" w611 {
          tunnel: w609 -> [w621 w624]
          tunnel: [w620 w623] -> w602
          tunnel: w598 -> [w618 _]
          frame "on", Default {
            w619 = u16 1 items=["Continuous", "Pulsed"] ("sweep method")
            n171 = Fract/Exp String To Number(string=w618) -> (number=w616:dbl[])  [unwired: 3 in, 1 out]
            n172 = Index Array(array=w616, index #1=0 ("Index")) -> (element #1=w615:dbl, element #2=w614:dbl, element #3=w613:dbl)  [unwired: 2 in]
            n173 = Bundle By Name(cluster=w621, "sweep method"=w619, "Pulse period"=w615, "Base voltage"=w614, "Pulse width"=w613) -> (w620:T5)
          }
          frame "off" {
            w622 = u16 0 items=["Continuous", "Pulsed"] ("sweep method")
            n174 = Bundle By Name(cluster=w624, "sweep method"=w622) -> (w623:T5)
          }
        }
      }
      frame "gaterangemode" {
        n175 = Delete From Array(array=w638, index=0 ("Index")) -> (deleted portion=w639:string)  [unwired: 1 in, 1 out]
        n176 = case shown="\"f\"" w639 {
          tunnel: [w641 w642 w643] -> w628
          frame "a", Default {
            w641 = u16 0 items=["Auto", "Limited", "Fixed"] ("Gate Range\nmode 2")
          }
          frame "f" {
            w642 = u16 2 items=["Auto", "Limited", "Fixed"] ("Gate Range\nmode 2")
          }
          frame "l" {
            w643 = u16 1 items=["Auto", "Limited", "Fixed"] ("Gate Range\nmode 2")
          }
        }
      }
      frame "gaterange" {
        (unwired) u8 11 items=["10fA  ", "100fA  ", "1nA  ", "10nA", "100nA", "1uA", "10uA", "100uA", "1mA", "10mA", "100mA", "1A"] ("Gate Range 2")
        n177 = Delete From Array(array=w664, index=0 ("Index")) -> (deleted portion=w654:string)  [unwired: 1 in, 1 out]
        n178 = Scan Value(string=w654, format string="") -> (value=w652:dbl)  [unwired: 1 in, 1 out]
        n179 = Logarithm Base 10(1:w652) -> (0:w651:dbl)
        n180 = Round To Nearest(number=w651) -> (nearest integer value=w650:dbl)
        n181 = Add(x=w650, y=11.0) -> (x+y=w648:dbl)
        n182 = To Unsigned Byte Integer(number=w648) -> (unsigned 8bit integer=w647:u8)
      }
      frame "drainrange" {
        (unwired) u8 11 items=["10fA  ", "100fA  ", "1nA  ", "10nA", "100nA", "1uA", "10uA", "100uA", "1mA", "10mA", "100mA", "1A"] ("Gate Range 2")
        n183 = Delete From Array(array=w686, index=0 ("Index")) -> (deleted portion=w677:string)  [unwired: 1 in, 1 out]
        n184 = Scan Value(string=w677, format string="") -> (value=w675:dbl)  [unwired: 1 in, 1 out]
        n185 = Logarithm Base 10(1:w675) -> (0:w674:dbl)
        n186 = Round To Nearest(number=w674) -> (nearest integer value=w673:dbl)
        n187 = Add(x=w673, y=11.0) -> (x+y=w671:dbl)
        n188 = To Unsigned Byte Integer(number=w671) -> (unsigned 8bit integer=w670:u8)
      }
      frame "drainrangemode" {
        n189 = Delete From Array(array=w701, index=0 ("Index")) -> (deleted portion=w702:string)  [unwired: 1 in, 1 out]
        n190 = case shown="\"f\"" w702 {
          tunnel: [w704 w705 w706] -> w691
          frame "a", Default {
            w704 = u16 0 items=["Auto", "Limited", "Fixed"] ("Gate Range\nmode 2")
          }
          frame "f" {
            w705 = u16 2 items=["Auto", "Limited", "Fixed"] ("Gate Range\nmode 2")
          }
          frame "l" {
            w706 = u16 1 items=["Auto", "Limited", "Fixed"] ("Gate Range\nmode 2")
          }
        }
      }
      frame "Error", Default {
      }
      frame "logfile" {
        n191 = Number To Decimal String(number=w723) -> (decimal integer string=w758:string)  [unwired: 1 in]
        n192 = Concatenate Strings(w757, "logfile" ("Substring"), w758, w721, ".txt" ("Substring")) -> (w755:string)
        n193 = String To Path(string=w755) -> (path=w728:path)
        n194 = Unbundle(w754) -> ("integration time"=w753:u32, "Short/Long integration time"=w752:dbl, "hold time (sec)"=w751:dbl, "delay time (sec)"=w750:dbl, "Step Time (0 disables)"=w749:dbl, "sweep method"=w748:u16, "Pulse period"=w747:dbl, "Base voltage"=w746:dbl, "Pulse width"=w745:dbl)
        n195 = Build Array(w753, w752, w751, w750, w749, w748, w747, w746, w745, w739, w740, w741, w742, w743, w744) -> (w732:dbl[])
        n196 = Insert Into Array(array=dbl[][] [] ("Input Array"), new element=w732) -> (w731:dbl[][])  [unwired: 2 in]
        n197 = call <vilib>:"compatOverwrite.vi"("overwrite (F)"=TRUE) -> ("overwrite?"=w726:T7)
        n198 = Open/Create/Replace File(file path (use dialog)=w728, error in=w730, operation (0:open)=w726) -> (refnum out=w736:refnum<file>, error out=w735:errorcluster)  [unwired: 3 in, 1 out]
        n199 = call "4155C Write array to file.vi"("Byte Stream File Refnum"=w736, "Header"=string[] ["Int Time", "Short/Long Itime", "Hold time", "Delay time", "Step time", "Sweep method", "Pulse period", "Base Voltage", "Pulse width", "Drain compliance", "Gate compliance", "Gate range mode", "Gate range", "S/D range mode", "S/D range"], "Data Array"=w731, "error in (no error)"=w735) -> ("dup refnum"=w738:refnum<file>, "error out"=w737:errorcluster)  [unwired: 1 in]
        n200 = Close File(refnum=w738, error in=w737) -> (error out=w729:errorcluster)  [unwired: 1 out]
      }
      frame "sample" {
        n201 = Number To Decimal String(number=w763) -> (decimal integer string=w811:string)  [unwired: 1 in]
        n202 = Fract/Exp String To Number(string=w808) -> (number=w769:dbl[])  [unwired: 3 in, 1 out]
        n203 = Concatenate Strings(w786, "-sample-" ("Substring"), w811, w761, ".txt" ("Substring")) -> (w809:string)
        n204 = String To Path(string=w809) -> (path=w790:path)
        n205 = Index Array(array=w769, index=0 ("Index")) -> (element=w806:dbl)
        n206 = Index Array(array=w769, index=2 ("Index")) -> (element=w802:dbl)
        n207 = Index Array(array=w769, index=3 ("Index")) -> (element=w771:dbl)
        n208 = Index Array(array=w769, index=4 ("Index")) -> (element=w768:dbl)
        n209 = call "4155C Config Sampling Measurements.vi"("Sampling interval"=w768, "Sample time"=w771, "Display on/off"=TRUE, "Timings"=w777, "Num Points"=w802, "error in (no error)"=w813, "Drain Compliance"=w812, "Gate Compliance"=w787, "VISA session"=w814) -> ("error out"=w815:errorcluster, "dup VISA resource name"=w816:refnum<visa-resource-name>)  [unwired: 1 in]
        n210 = Index Array(array=w769, index=1 ("Index")) -> (element=w803:dbl)
        n211 = call "4155C Take Sample.vi"("Emergency Stop"=w783, "error in (no error)"=w815, "Vd"=w803, "Vg"=w806, "VISA resource name in"=w816) -> ("error out"=w781:errorcluster, "Id"=w818:dbl[], "Ig"=w792:dbl[], "VISA Resource Name out"=w779:refnum<visa-resource-name>, "Is"=w817:dbl[], "Time"=w796:dbl[])  [unwired: 1 in]
        n212 = Insert Into Array(array=dbl[][] [] ("Input Array"), new element=w796) -> (w795:dbl[][])  [unwired: 2 in]
        n213 = Insert Into Array(array=w795, new element=w792) -> (w794:dbl[][])  [unwired: 2 in]
        n214 = Insert Into Array(array=w794, new element=w818) -> (w793:dbl[][])  [unwired: 2 in]
        n215 = VISA Write(VISA resource name=w779, write buffer=":DISP ON" ("write buffer (\"\")"), error in (no error)=w781) -> (VISA resource name out=w778:refnum<visa-resource-name>, error out=w780:errorcluster)  [unwired: 1 out]
        n216 = Insert Into Array(array=w793, new element=w817) -> (w785:dbl[][])  [unwired: 2 in]
        n217 = Transpose 2D Array(2D array=w785) -> (transposed array=w784:dbl[][])
        n218 = call <vilib>:"compatOverwrite.vi"("overwrite (F)"=TRUE) -> ("overwrite?"=w766:T7)
        n219 = Open/Create/Replace File(file path (use dialog)=w790, error in=w780, operation (0:open)=w766) -> (refnum out=w799:refnum<file>, error out=w798:errorcluster)  [unwired: 3 in, 1 out]
        n220 = call "4155C Write array to file.vi"("Byte Stream File Refnum"=w799, "Header"=string[] ["Time /s", "Ig /A", "Id /A", "Is /A"], "Data Array"=w784, "error in (no error)"=w798) -> ("dup refnum"=w801:refnum<file>, "error out"=w800:errorcluster)  [unwired: 1 in]
        n221 = Close File(refnum=w801, error in=w800) -> (error out=w788:errorcluster)  [unwired: 1 out]
      }
      frame "samplei" {
        n222 = Number To Decimal String(number=w821) -> (decimal integer string=w873:string)  [unwired: 1 in]
        n223 = Fract/Exp String To Number(string=w870) -> (number=w837:dbl[])  [unwired: 3 in, 1 out]
        n224 = Concatenate Strings(w852, "-samplei-" ("Substring"), w873, w820, ".txt" ("Substring")) -> (w871:string)
        n225 = String To Path(string=w871) -> (path=w855:path)
        n226 = Index Array(array=w837, index=4 ("Index")) -> (element=w831:dbl)
        n227 = Index Array(array=w837, index=3 ("Index")) -> (element=w832:dbl)
        n228 = Index Array(array=w837, index=1 ("Index")) -> (element=w834:dbl)
        n229 = Index Array(array=w837, index=0 ("Index")) -> (element=w835:dbl)
        n230 = Index Array(array=w837, index=2 ("Index")) -> (element=w833:dbl)
        n231 = call "4155C Config SamplingI Measurements.vi"("Sample time"=w833, "Display on/off"=TRUE, "Timings"=w844, "Num Points"=w834, "error in (no error)"=w875, "Sampling interval"=w832, "VISA session"=w876) -> ("error out"=w877:errorcluster, "dup VISA resource name"=w878:refnum<visa-resource-name>)  [unwired: 3 in]
        n232 = call "4155C Take SampleI.vi"("Emergency Stop"=w849, "error in (no error)"=w877, "Idg 2"=w835, "Vdg compliance 2"=w831, "VISA resource name in"=w878) -> ("error out"=w847:errorcluster, "Idg"=w880:dbl[], "Vdg"=w857:dbl[], "VISA Resource Name out"=w845:refnum<visa-resource-name>, "Is"=w879:dbl[], "Time"=w861:dbl[])  [unwired: 1 in]
        n233 = Insert Into Array(array=dbl[][] [] ("Input Array"), new element=w861) -> (w860:dbl[][])  [unwired: 2 in]
        n234 = Insert Into Array(array=w860, new element=w857) -> (w859:dbl[][])  [unwired: 2 in]
        n235 = Insert Into Array(array=w859, new element=w880) -> (w858:dbl[][])  [unwired: 2 in]
        n236 = VISA Write(VISA resource name=w845, write buffer=":DISP ON" ("write buffer (\"\")"), error in (no error)=w847) -> (VISA resource name out=w830:refnum<visa-resource-name>, error out=w846:errorcluster)  [unwired: 1 out]
        n237 = Insert Into Array(array=w858, new element=w879) -> (w851:dbl[][])  [unwired: 2 in]
        n238 = Transpose 2D Array(2D array=w851) -> (transposed array=w850:dbl[][])
        n239 = call <vilib>:"compatOverwrite.vi"("overwrite (F)"=TRUE) -> ("overwrite?"=w825:T7)
        n240 = Open/Create/Replace File(file path (use dialog)=w855, error in=w846, operation (0:open)=w825) -> (refnum out=w864:refnum<file>, error out=w863:errorcluster)  [unwired: 3 in, 1 out]
        n241 = call "4155C Write array to file.vi"("Byte Stream File Refnum"=w864, "Header"=string[] ["Time /s", "Vdg /V", "Idg /A", "Is /A"], "Data Array"=w850, "error in (no error)"=w863) -> ("dup refnum"=w866:refnum<file>, "error out"=w865:errorcluster)  [unwired: 1 in]
        n242 = Close File(refnum=w866, error in=w865) -> (error out=w828:errorcluster)  [unwired: 1 out]
        n243 = VISA Write(VISA resource name=w830, write buffer=";:PAGE:SCON:STAN OFF;:PAGE:CHAN:VSU2:DIS;" ("write buffer (\"\")"), error in (no error)=w828) -> (VISA resource name out=w826:refnum<visa-resource-name>, error out=w827:errorcluster)  [unwired: 1 out]
      }
      frame "#" {
        n244 = VISA Write(VISA resource name=w888, write buffer=":DISP ON" ("write buffer (\"\")"), error in (no error)=w887) -> (VISA resource name out=w886:refnum<visa-resource-name>, error out=w885:errorcluster)  [unwired: 1 out]
      }
      frame "stressV" {
        n245 = Number To Decimal String(number=w899) -> (decimal integer string=w940:string)  [unwired: 1 in]
        n246 = Fract/Exp String To Number(string=w937) -> (number=w910:dbl[])  [unwired: 3 in, 1 out]
        n247 = Concatenate Strings(w924, "-stressV-" ("Substring"), w940, w898, ".txt" ("Substring")) -> (w938:string)
        n248 = String To Path(string=w938) -> (path=w928:path)
        n249 = Index Array(array=w910, index=3 ("Index")) -> (element=w907:dbl)
        n250 = Index Array(array=w910, index=1 ("Index")) -> (element=w905:dbl)
        n251 = Index Array(array=w910, index=0 ("Index")) -> (element=w904:dbl)
        n252 = Index Array(array=w910, index=4 ("Index")) -> (element=w909:dbl)
        n253 = Index Array(array=w910, index=2 ("Index")) -> (element=w906:dbl)
        n254 = call "4155C Config V Stress.vi"("VISA session"=w943, "ID compliance"=w907, "VD"=w905, "VG"=w904, "IG compliance"=w906, "error in (no error)"=w942, "Display on/off"=TRUE) -> ("dup VISA resource name"=w945:refnum<visa-resource-name>, "error out"=w944:errorcluster)
        n255 = call "4155C Apply Stress.vi"("error in (no error)"=w944, "Duration"=w909, "Emergency Stop"=w923, "VISA resource name in"=w945) -> ("error out"=w921:errorcluster, "VISA Resource Name out"=w919:refnum<visa-resource-name>)
        n256 = VISA Write(VISA resource name=w919, write buffer=":DISP ON" ("write buffer (\"\")"), error in (no error)=w921) -> (VISA resource name out=w918:refnum<visa-resource-name>, error out=w920:errorcluster)  [unwired: 1 out]
        n257 = call <vilib>:"compatOverwrite.vi"("overwrite (F)"=TRUE) -> ("overwrite?"=w903:T7)
        n258 = Open/Create/Replace File(file path (use dialog)=w928, error in=w920, operation (0:open)=w903) -> (refnum out=w931:refnum<file>, error out=w930:errorcluster)  [unwired: 3 in, 1 out]
        n259 = call "4155C Write array to file.vi"("Byte Stream File Refnum"=w931, "Header"=string[] ["V stress completed successfully", ""], "error in (no error)"=w930) -> ("dup refnum"=w933:refnum<file>, "error out"=w932:errorcluster)  [unwired: 2 in]
        n260 = Close File(refnum=w933, error in=w932) -> (error out=w926:errorcluster)  [unwired: 1 out]
      }
      frame "stressI" {
        n261 = Number To Decimal String(number=w948) -> (decimal integer string=w985:string)  [unwired: 1 in]
        n262 = Fract/Exp String To Number(string=w982) -> (number=w957:dbl[])  [unwired: 3 in, 1 out]
        n263 = Concatenate Strings(w969, "-stressI-" ("Substring"), w985, w947, ".txt" ("Substring")) -> (w983:string)
        n264 = String To Path(string=w983) -> (path=w973:path)
        n265 = Index Array(array=w957, index=1 ("Index")) -> (element=w953:dbl)
        n266 = Index Array(array=w957, index=0 ("Index")) -> (element=w954:dbl)
        n267 = call "4155C Config I Stress.vi"("VISA session"=w988, "IDG"=w954, "VDG compliance"=w953, "error in (no error)"=w987, "Display on/off"=TRUE) -> ("dup VISA resource name"=w990:refnum<visa-resource-name>, "error out"=w989:errorcluster)
        n268 = Index Array(array=w957, index=2 ("Index")) -> (element=w955:dbl)
        n269 = call "4155C Apply Stress.vi"("error in (no error)"=w989, "Duration"=w955, "Emergency Stop"=w968, "VISA resource name in"=w990) -> ("error out"=w966:errorcluster, "VISA Resource Name out"=w964:refnum<visa-resource-name>)
        n270 = VISA Write(VISA resource name=w964, write buffer=":DISP ON" ("write buffer (\"\")"), error in (no error)=w966) -> (VISA resource name out=w963:refnum<visa-resource-name>, error out=w965:errorcluster)  [unwired: 1 out]
        n271 = call <vilib>:"compatOverwrite.vi"("overwrite (F)"=TRUE) -> ("overwrite?"=w952:T7)
        n272 = Open/Create/Replace File(file path (use dialog)=w973, error in=w965, operation (0:open)=w952) -> (refnum out=w976:refnum<file>, error out=w975:errorcluster)  [unwired: 3 in, 1 out]
        n273 = call "4155C Write array to file.vi"("Byte Stream File Refnum"=w976, "Header"=string[] ["I stress completed successfully", ""], "error in (no error)"=w975) -> ("dup refnum"=w978:refnum<file>, "error out"=w977:errorcluster)  [unwired: 2 in]
        n274 = Close File(refnum=w978, error in=w977) -> (error out=w971:errorcluster)  [unwired: 1 out]
      }
      frame "vsu2pulse" {
        n275 = Number To Decimal String(number=w993) -> (decimal integer string=w1028:string)  [unwired: 1 in]
        n276 = Fract/Exp String To Number(string=w1025) -> (number=w1001:dbl[])  [unwired: 3 in, 1 out]
        n277 = Concatenate Strings(w1013, "-vsu2-" ("Substring"), w1028, w992, ".txt" ("Substring")) -> (w1026:string)
        n278 = String To Path(string=w1026) -> (path=w1017:path)
        n279 = Index Array(array=w1001, index=1 ("Index")) -> (element=w1000:dbl)
        n280 = Index Array(array=w1001, index=0 ("Index")) -> (element=w998:dbl)
        n281 = call "4155C Config VSU2 Stress.vi"("error in (no error)"=w1030, "VSU2"=w998, "Display on/off"=TRUE, "VISA session"=w1031) -> ("error out"=w1032:errorcluster, "dup VISA resource name"=w1033:refnum<visa-resource-name>)
        n282 = call "4155C Apply Stress.vi"("error in (no error)"=w1032, "Duration"=w1000, "Emergency Stop"=w1012, "VISA resource name in"=w1033) -> ("error out"=w1010:errorcluster, "VISA Resource Name out"=w1008:refnum<visa-resource-name>)
        n283 = VISA Write(VISA resource name=w1008, write buffer=":DISP ON" ("write buffer (\"\")"), error in (no error)=w1010) -> (VISA resource name out=w1007:refnum<visa-resource-name>, error out=w1009:errorcluster)  [unwired: 1 out]
        n284 = call <vilib>:"compatOverwrite.vi"("overwrite (F)"=TRUE) -> ("overwrite?"=w997:T7)
        n285 = Open/Create/Replace File(file path (use dialog)=w1017, error in=w1009, operation (0:open)=w997) -> (refnum out=w1020:refnum<file>, error out=w1019:errorcluster)  [unwired: 3 in, 1 out]
        n286 = call "4155C Write array to file.vi"("Byte Stream File Refnum"=w1020, "Header"=string[] ["VSU2 pulse completed successfully", ""], "error in (no error)"=w1019) -> ("dup refnum"=w1022:refnum<file>, "error out"=w1021:errorcluster)  [unwired: 2 in]
        n287 = Close File(refnum=w1022, error in=w1021) -> (error out=w1015:errorcluster)  [unwired: 1 out]
      }
      frame "sample-fpp" {
        w1047 = string[] ["Time /s", "Id VgVd /A", "Ig VgVd /A", "Vp1 VgVd /V", "Vp2 VgVd /V"] ("Header")
        w1051 = "%d" ("format string")
        n288 = Number To Decimal String(number=w1036) -> (decimal integer string=w1099:string)  [unwired: 1 in]
        n289 = Fract/Exp String To Number(string=w1096) -> (number=w1084:dbl[])  [unwired: 3 in, 1 out]
        n290 = Concatenate Strings(w1090, "-samplefpp-" ("Substring"), w1099, w1035, ".txt" ("Substring")) -> (w1097:string)
        n291 = String To Path(string=w1097) -> (path=w1059:path)
        n292 = Index Array(array=w1084, index=0 ("Index")) -> (element=w1045:dbl)
        n293 = Index Array(array=w1084, index=1 ("Index")) -> (element=w1044:dbl)
        n294 = Index Array(array=w1084, index=2 ("Index")) -> (element=w1092:dbl)
        n295 = Index Array(array=w1084, index=3 ("Index")) -> (element=w1082:dbl)
        n296 = call "4155C Config Sampling Measurements FPP.vi"("VISA session"=w1102, "Num Points"=w1092, "Vg"=w1045, "Display on/off"=TRUE, "Gate Compliance"=w1091, "Drain Compliance"=w1100, "Standby"="Standby", "error in (no error)"=w1101, "Timings"=w1089, "Vd"=w1044, "Sample time"=w1082) -> ("dup VISA resource name"=w1061:refnum<visa-resource-name>, "error out"=w1060:errorcluster)  [unwired: 3 in]
        n297 = Number To Decimal String(number=w1045) -> (decimal integer string=w1071:string)  [unwired: 1 in]
        n298 = call "4155C Take Sample FPP.vi"("VISA resource name in"=w1061, "error in (no error)"=w1060, "Emergency Stop"=w1062) -> ("Time"=w1066:dbl[], "Vp1"=w1076:dbl[], "VISA Resource Name out"=w1042:refnum<visa-resource-name>, "Ig"=w1064:dbl[], "Id"=w1065:dbl[], "Vp2"=w1074:dbl[], "error out"=w1063:errorcluster)  [unwired: 10 in]
        n299 = Insert Into Array(array=dbl[][] [] ("Input Array"), new element=w1066) -> (w1080:dbl[][])  [unwired: 2 in]
        n300 = Number To Decimal String(number=w1044) -> (decimal integer string=w1069:string)  [unwired: 1 in]
        n301 = Insert Into Array(array=w1080, new element=w1065) -> (w1079:dbl[][])  [unwired: 2 in]
        n302 = Concatenate Strings("(Vg = " ("Substring"), w1071, "V, Vd = " ("Substring"), w1069, "V)" ("Substring")) -> (w1067:string)
        n303 = Insert Into Array(array=w1079, new element=w1064) -> (w1078:dbl[][])  [unwired: 2 in]
        n304 = Insert Into Array(array=w1078, new element=w1076) -> (w1075:dbl[][])  [unwired: 2 in]
        n305 = Insert Into Array(array=w1075, new element=w1074) -> (w1043:dbl[][])  [unwired: 2 in]
        n306 = call <vilib>:"compatOverwrite.vi"("overwrite (F)"=TRUE) -> ("overwrite?"=w1040:T7)
        n307 = Open/Create/Replace File(file path (use dialog)=w1059, error in=w1063, operation (0:open)=w1040) -> (refnum out=w1056:refnum<file>, error out=w1057:errorcluster)  [unwired: 3 in, 1 out]
        n308 = Array To Spreadsheet String(array=w1047, 3:w1051) -> (spreadsheet string=w1053:string)  [unwired: 1 in]
        n309 = Transpose 2D Array(2D array=w1043) -> (transposed array=w1073:dbl[][])
        n310 = Search and Replace String(replace all?=TRUE ("replace all? (F)"), input string=w1053, search string="VgVd", replace string=w1067) -> (result string=w1049:string)  [unwired: 4 in, 3 out]
        n311 = Spreadsheet String To Array(format string=w1051, spreadsheet string=w1049, array type (2D Dbl)=w1047) -> (array=w1048:string[])  [unwired: 1 in]
        n312 = call "4155C Write array to file.vi"("Byte Stream File Refnum"=w1056, "Header"=w1048, "Data Array"=w1073, "error in (no error)"=w1057) -> ("dup refnum"=w1054:refnum<file>, "error out"=w1055:errorcluster)  [unwired: 1 in]
        n313 = Close File(refnum=w1054, error in=w1055) -> (error out=w1041:errorcluster)  [unwired: 1 out]
      }
      frame "resample-fpp" {
        w1118 = string[] ["Time /s", "Id VgVd /A", "Ig VgVd /A", "Vp1 VgVd /V", "Vp2 VgVd /V"] ("Header")
        w1122 = "%d" ("format string")
        n314 = Number To Decimal String(number=w1104) -> (decimal integer string=w1162:string)  [unwired: 1 in]
        n315 = Fract/Exp String To Number(string=w1159) -> (number=w1111:dbl[])  [unwired: 3 in, 1 out]
        n316 = Concatenate Strings(w1155, "-resamplefpp-" ("Substring"), w1162, w1105, ".txt" ("Substring")) -> (w1160:string)
        n317 = String To Path(string=w1160) -> (path=w1130:path)
        n318 = Index Array(array=w1111, index=0 ("Index")) -> (element=w1117:dbl)
        n319 = Index Array(array=w1111, index=1 ("Index")) -> (element=w1116:dbl)
        n320 = Number To Decimal String(number=w1117) -> (decimal integer string=w1140:string)  [unwired: 1 in]
        n321 = call "4155C Take Sample FPP.vi"("VISA resource name in"=w1113, "error in (no error)"=w1112, "Emergency Stop"=w1131) -> ("Time"=w1135:dbl[], "Vp1"=w1145:dbl[], "VISA Resource Name out"=w1115:refnum<visa-resource-name>, "Ig"=w1133:dbl[], "Id"=w1134:dbl[], "Vp2"=w1143:dbl[], "error out"=w1132:errorcluster)  [unwired: 10 in]
        n322 = Insert Into Array(array=dbl[][] [] ("Input Array"), new element=w1135) -> (w1149:dbl[][])  [unwired: 2 in]
        n323 = Number To Decimal String(number=w1116) -> (decimal integer string=w1138:string)  [unwired: 1 in]
        n324 = Insert Into Array(array=w1149, new element=w1134) -> (w1148:dbl[][])  [unwired: 2 in]
        n325 = Concatenate Strings("(Vg = " ("Substring"), w1140, "V, Vd = " ("Substring"), w1138, "V)" ("Substring")) -> (w1136:string)
        n326 = Insert Into Array(array=w1148, new element=w1133) -> (w1147:dbl[][])  [unwired: 2 in]
        n327 = Insert Into Array(array=w1147, new element=w1145) -> (w1144:dbl[][])  [unwired: 2 in]
        n328 = Insert Into Array(array=w1144, new element=w1143) -> (w1110:dbl[][])  [unwired: 2 in]
        n329 = call <vilib>:"compatOverwrite.vi"("overwrite (F)"=TRUE) -> ("overwrite?"=w1109:T7)
        n330 = Open/Create/Replace File(file path (use dialog)=w1130, error in=w1132, operation (0:open)=w1109) -> (refnum out=w1127:refnum<file>, error out=w1128:errorcluster)  [unwired: 3 in, 1 out]
        n331 = Array To Spreadsheet String(array=w1118, 3:w1122) -> (spreadsheet string=w1124:string)  [unwired: 1 in]
        n332 = Transpose 2D Array(2D array=w1110) -> (transposed array=w1142:dbl[][])
        n333 = Search and Replace String(replace all?=TRUE ("replace all? (F)"), input string=w1124, search string="VgVd", replace string=w1136) -> (result string=w1120:string)  [unwired: 4 in, 3 out]
        n334 = Spreadsheet String To Array(format string=w1122, spreadsheet string=w1120, array type (2D Dbl)=w1118) -> (array=w1119:string[])  [unwired: 1 in]
        n335 = call "4155C Write array to file.vi"("Byte Stream File Refnum"=w1127, "Header"=w1119, "Data Array"=w1142, "error in (no error)"=w1128) -> ("dup refnum"=w1125:refnum<file>, "error out"=w1126:errorcluster)  [unwired: 1 in]
        n336 = Close File(refnum=w1125, error in=w1126) -> (error out=w1114:errorcluster)  [unwired: 1 out]
      }
      frame "serial" {
        n337 = Index Array(array=w1167, index=0 ("Index")) -> (element=w1166:string)
        n338 = call "Serial write and read v0.4.vi"("Termination char\n(0xA = '\\n' = LF)\n(0xD = '\\r' = CR)"="Termination char\n(0xA = '\\n' = LF)\n(0xD = '\\r' = CR)", "Enable Termination\nChar (T)"="Enable Termination\nChar (T)", "parity"="parity", "stop bits"="stop bits", "string to write"=w1166, "flow control"="flow control", "byte count"="byte count", "Serial Settings:Serial End Mode for Reads"="Serial End Mode for Reads", "Timeout (ms)"="Timeout (ms)", "error in (no error)"=w1172, "VISA resource name"="VISA resource name", "baud rate"="baud rate", "data bits"="data bits") -> ("read string"=→"Serial port output":string, "error out"=w1171:errorcluster)  [unwired: 1 in]
      }
    }
    n339 = Build Array("Time /s" ("element"), "Id max /A" ("VAR2 Name"), "Id min /A" ("VAR2 Name")) -> (w68:string[])
    n340 = Build Array(w63, w62, w54) -> (w61:dbl[][])
    n341 = Transpose 2D Array(2D array=w61) -> (transposed array=w60:dbl[][])
    n342 = Concatenate Strings(w59, "-Ion-Ioff", ".txt" ("Suffix")) -> (w76:string)
    n343 = Array To Spreadsheet String(array=w68, 3:"" ("format string")) -> (spreadsheet string=w67:string)  [unwired: 1 in]
    n344 = Array To Spreadsheet String(array=w60, 3:"%e" ("format string")) -> (spreadsheet string=w66:string)  [unwired: 1 in]
    n345 = String To Path(string=w76) -> (path=w75:path)
    n346 = Build Array(w67, w66) -> (w65:string[])
    n347 = Write to Text File(file (use dialog)=w75, text=w65, error in=w57) -> (refnum out=w77:refnum<file>, error out=w64:errorcluster)  [unwired: 1 in, 1 out]
    n348 = Close File(refnum=w77, error in=w64) -> (error out=w56:errorcluster)  [unwired: 1 out]
    "Line running" <- w87
    "Total lines" <- w86
  }
  "error out" <- w7
